vi "FocalMainV1.vi"() -> ()   [LabVIEW 2018]
uses:
  Clusters/FileDataChannel.ctl
  Clusters/BladePitchMode.ctl
  Clusters/GenMode.ctl
  Clusters/IndicatorScale.ctl
  Clusters/SimulationConstants.ctl
  <vilib>/Platform/TimedLoop/XDataNode/timing_clust.ctl
  <vilib>/Platform/TimedLoop/XDataNode/nitl_modes.ctl
  <vilib>/Platform/TimedLoop/XDataNode/wakeup.ctl
  Clusters/IOSignals.ctl
  Clusters/ArrayPairs.ctl
  Clusters/SwapArrayCluster.ctl
  Clusters/ElmoState.ctl
  Clusters/PLCSignals.ctl
  Clusters/CtrlSignals.ctl
  Clusters/ScalingEnum.ctl
  Clusters/RoscoParams.ctl
  Clusters/GenCtrl.ctl
  Clusters/PitchCtrl.ctl
  <vilib>/Utility/file.llb/Read Delimited Spreadsheet (DBL).vi
  SubVIs/InsertIntoArray_v2.vi
  <vilib>/platform/TimedLoop/XDataNode/XDataNode.xnode
  <vilib>/Platform/TimedLoop/XDataNode/XDNodeRunTimeDep.lvlib
  <resource>/objmgr/IndComECAT.rc
  usr/local/lib/libCallROSCO.so
panel:
  out "towerBotMy":dbl
  out "Current Setting":dbl[](array[numeric])
  in  "Commit":bool
  in  "Fan Setpoint (%)":dbl format="%#_13g"
  in  "Clear Faults":bool
  in  "Enable Fans":bool
  in  "Turn Fans On":bool
  out "Fy":dbl format="%#_5g"
  out "Fx":dbl
  out "PLC read errors":string
  out "PLC read/write late?":bool
  out "PLC Read Error":bool
  out "Axis 3 Homing":bool
  out "Axis 2 Homing":bool
  out "Axis 1 Homing":bool
  in  "Home Blades (x3)":bool
  out "Axis 3 Homed":bool
  out "Axis 2 Homed":bool
  out "Axis 1 Homed":bool
  out "SimulationConst":T1={"nGear"=1.0, "rotorRadius"=120.0, "numBlades"=3, "scaleFactor"=70.0, "roscoInitMinSpeed_rad_s"=0.5, "roscoInitMinTorqueFS_Nm"=1000000.0, "beckhoff24BitExt"=7812500, "torqueCellFullV"=5.0, "torqueCellFullNm"=2.0, "torqueCellELM3148V"=10.0, "nacelleAccELM3604V"=1.25, "nacelleAccScaleX"=0.0673, "nacelleAccOfstX"=0.0055, "nacelleAccScaleY"=0.0672, "nacelleAccOfstY"=0.0049, "nacelleAccScaleZ"=0.0677, "nacelleAccOfstZ"=0.0087, "cyberGearRatio"=0.5, "cyberLinesPerRev"=0.5, "cyberRatedTorque"=0.5, "towerTopForceScale"=0.5, "towerTopTorqueScale"=0.5, "plcSetpointScaling_norm2VFD"=0.5, "towerBotScaleMy_Nm_V"=0.5, "towerBotOfstMy_Nm"=0.5, "towerTopScaleXaxis_N_V"=0.5, "towerTopOfstXaxis_N"=0.5, "towerTopScaleYaxis_N_V"=0.5, "towerTopOfstYaxis_N"=0.5} {"beckhoff24BitExt" format="%x"}
  out "nacelleAccZ (m/s2)":dbl
  out "nacelleAccY (m/s2)":dbl
  out "nacelleAccX (m/s2)":dbl
  out "Disk > 2GB free?":bool
  out "Current OP mode":T2
  in  "IndicatorScale":T3
  in  "DISCON.IN file":string="DISCON-UMaineSemi.IN"
  in  "Cp/Ct/Cq file":string="Cp_Ct_Cq.IEA15MW.txt"
  out "Torque sine period FS (Nm)":dbl format="%.2g"
  out "Torque sine amp FS (Nm)":dbl format="%.2g"
  out "Torque sine mean FS (Nm)":dbl format="%.2g"
  out "Ramp time FS (s)":dbl format="%.2g"
  out "Ramp target vel FS (rpm)":dbl format="%.2g"
  out "Const. vel setpoint FS (rpm)":dbl format="%.2g"
  out "From File Vel FS (rpm)":dbl
  out "From File Pitch FS (deg)":dbl
  out "Exp time FS (s)":dbl format="%5.2f"
  in  "Commit get settings":bool
  out "Current OP mode":T4
  in  "Commit pitch settings":bool
  in  "Start / Stop Run":bool
  out "Speed Setpoint (rpm)":dbl(knob)=7.068579725455493e-05 scale=0.0..20.0
  out "Pitch Blade 3 (deg)":dbl
  out "Pitch Bade 2 (deg)":dbl
  out "Pitch Blade 1 (deg)":dbl
  out "Pitch Setpoint (deg)":dbl
  out "Setpoint file loaded":path
  in  "Setpoint file name":string="setpointsVelTestA.txt"
  out "Torque sine period MS (Nm)":dbl format="%.2g"
  out "Torque sine amp MS (Nm)":dbl format="%#.2g"
  in  "Torque sine period (s)":dbl=100.0
  in  "Torque sine amp (MNm)":dbl
  out "Torque sine mean MS (Nm)":dbl format="%.2g"
  in  "Torque mean (MNm)":dbl
  out "Ramp time MS (s)":dbl format="%.2g"
  out "Ramp target vel MS (rpm)":dbl format="%.2g"
  out "Const. vel setpoint MS (rpm)":dbl format="%.2g"
  in  "Ramp time (s)":dbl=100.0
  in  "Ramp target vel (rpm)":dbl=10.0
  in  "Const. vel (rpm)":dbl
  out "Current Const. (deg)":dbl
  in  "Next OP mode":T2
  in  "Next Const. (deg)":dbl=10.0
  in  "Next OP mode":T4
  in  "Wind Est. u(t=0)":dbl=5.0
  out "Exp. Time MS (s)":dbl format="%5.1f"
  out "Output file Name":string
  out "State logic late?":bool
  out "Axis 3 Fault":bool
  out "Axis 3 Warning":bool
  out "Axis 2 Fault":bool
  out "Axis 2 Warning":bool
  out "Axis 1 Fault":bool
  out "Axis 1 Warning":bool
  out "Axis 3 Operational":bool
  out "Axis 2 Operational":bool
  out "Axis 1 Operational":bool
  out "Pitch Axis 3 State":string
  out "Pitch Axis 2 State":string
  out "Pitch Axis 1 State":string
  in  "Clear Pitch Actuator Faults (x3)":bool
  in  "Enable Pitch Actuators (x3)":bool
  out "Generator Operational":bool
  in  "Clear Accelnet Faults":bool
  in  "Enable Accelnet":bool
  out "Generator Fault":bool
  out "Generator Warning":bool
  out "Main generator state":string
  out "Rosco Failed?":bool
  out "Torque Cell":dbl(knob) scale=0.0..25.0
  out "Actual Speed MS (rpm)":dbl(knob)=7.068579725455493e-05 scale=0.0..20.0
  in  "?":T5(tab)
  out "Generator Speed":dynamicdata(graph)
  out "Rotor Loads":dynamicdata(graph)
  out "Pitch":dynamicdata(graph)
  out "TSR":dynamicdata(graph)
  out "DISCON.IN Contents":string
  out "Rosco Interface Current Message":string
  out "ROSCO DISCON.In file used":string
  out "ROSCO CpCqCt File used":string
  out "ROSCO out file used":string
  out "Test sum":sgl
  out "error out":errorcluster
  out "aviFAIL":i32
  out "Rosco Interface First Message":string
  out "Rosco Setpoint (Nm) - MS":dbl(knob) scale=0.0..10.0
  out "OUT_ROTSP":dbl
  out "OUT_AEROTQ":dbl
  out "Rosco Pitch Setpoint (rad)":dbl(knob) scale=0.0..10.0
  out "WE ROSCO":dbl
  out "avrSWAP":sgl[](array[numeric])
  out "Setpoints":dbl[][](array[numeric])
  out "Time index":i32
  out "Loop duration (ms)":i64
  in  "Pitch Max Vel Change (rpm/min) - FS":dbl=10.0
  in  "Pitch Max Vel (rpm) - FS":dbl=1.0
  in  "Pitch Homing Vel  (rpm) - FS":dbl=0.3
  in  "Pitch P-Gain":dbl=5.0
  in  "Max Vel (rpm)  -FS":dbl=14.0
  in  "Velocity Ctrl P-Gain":dbl=0.14
  in  "Velocity Ctrl I-Gain":dbl=3.0
  in  "Torque Ctrl FF Gain":dbl=1.15
  in  "Torque Ctrl I-Gain":dbl=5.0
  in  "Torque Ctrl P-Gain":dbl=0.05
  in  "Max Torque (MNm) - FS":dbl=25.0
  out "Pitch axis 3 ctrl word":u16 format="%x"
  out "Pitch axis 2 ctrl word":u16 format="%x"
  out "RT Loop Duration":i64
  out "Control Mode - Main Gen":u8
  out "WriteSDO Abort - Main Gen":u32
  out "ReadSDO Abort - Main Gen":u32
  out "Gen ctrl word":u16 format="%x"
  out "Pitch axis 1 ctrl word":u16 format="%x"
  out "Graphics Update t (s)":dbl format="%.1f"
  out "Effective graphics rate (ms)":dbl format="%#.1f"
  out "WriteSDO Abort - Pitch 1":u32
  out "ReadSDO Abort - Pitch 1":u32
  out "Control Mode - Pitch 1":u8
  out "Torque RAW (V)":dbl
  out "Torque Sensor (Nm) - NOT scaled":dbl(knob) scale=-2.0..2.0
  out "Free GB disk":dbl
  out "WriteSDO Abort - Pitch 2":u32
  out "Control Mode - Pitch 2":u8
  out "ReadSDO Abort - Pitch 2":u32
  out "WriteSDO Abort - Pitch 3":u32
  out "Control Mode - Pitch 3":u8
  out "ReadSDO Abort - Pitch 3":u32
  out "MotorDemandTorque_Nm":dbl(knob) scale=-2.0..2.0
  out "MotorCurrentTorq (Nm)":dbl(knob) scale=-2.0..2.0
  out "Axis 1 HomePos (rad)":dbl
  out "Axis 2 HomePos (rad)":dbl
  out "Axis 3 HomePos (rad)":dbl
  out "TSR 2":dynamicdata(graph)
  out "Init error":errorcluster
  out "Torque Setpoint":dbl(knob) scale=0.0..35.0
  out "Power (MW)":dbl(slide) scale=0.0..10.0 scale format="%.2f"
  out "FIFO Loop Late?":bool
  in  "Base filename":string="rosco-tests"
  out "Writing":bool
  in  "?":T6
  out "#RT FIFO":u32
  in  "Stop LabVIEW":bool
  out "cRio Time(s)":dbl format="%6.1f"
  out "RT Loop Late?":bool
  # "FOCAL Campaign 1 - V1.0"
  # "ROSCO OK?"
  # "GENERATOR ENABLE"
  # "BLADE PITCH"
  # "WIND MACHINE CONTROL"
  # "EXPERIMENT CONTROL"
  # "GENERATOR SETPOINT CTRL"
  # "PITCH ACTUATORS CONTROL"
  # "Nacelle Acceleration"
  # "TowerTop 3DOF"
  # "Blade1"
  # "Blade2"
  # "Blade3"
  # "Current values"
  # "Operational"
  # "Enter NEXT values (FS)"
  # "FS"
  # "MS"
  # "Homing"
  # "Homed"
  # "Warning"
  # "Error"
  # "TowerBot My"
  # "Fan 1"
  # "Time"
  # "Pitch"
  # "Vel"
  # "Fan 20"
  # "Fan 30"
  # "Fan 10"
  # "PI for Torque Ctrl"
  # "PI for Velocity Ctrl"
  # "PI for Pitch Ctrl"
  # "Main Gen Limits"
  # "Pitch limits"
  # "PITCH AXIS 1"
  # "PITCH AXIS 2"
  # "PITCH AXIS 3"
  # "TOWER TOP 6DOF"
  # "SYSTEM"
  # "GENERATOR"
  # "TORQUE SENSOR"
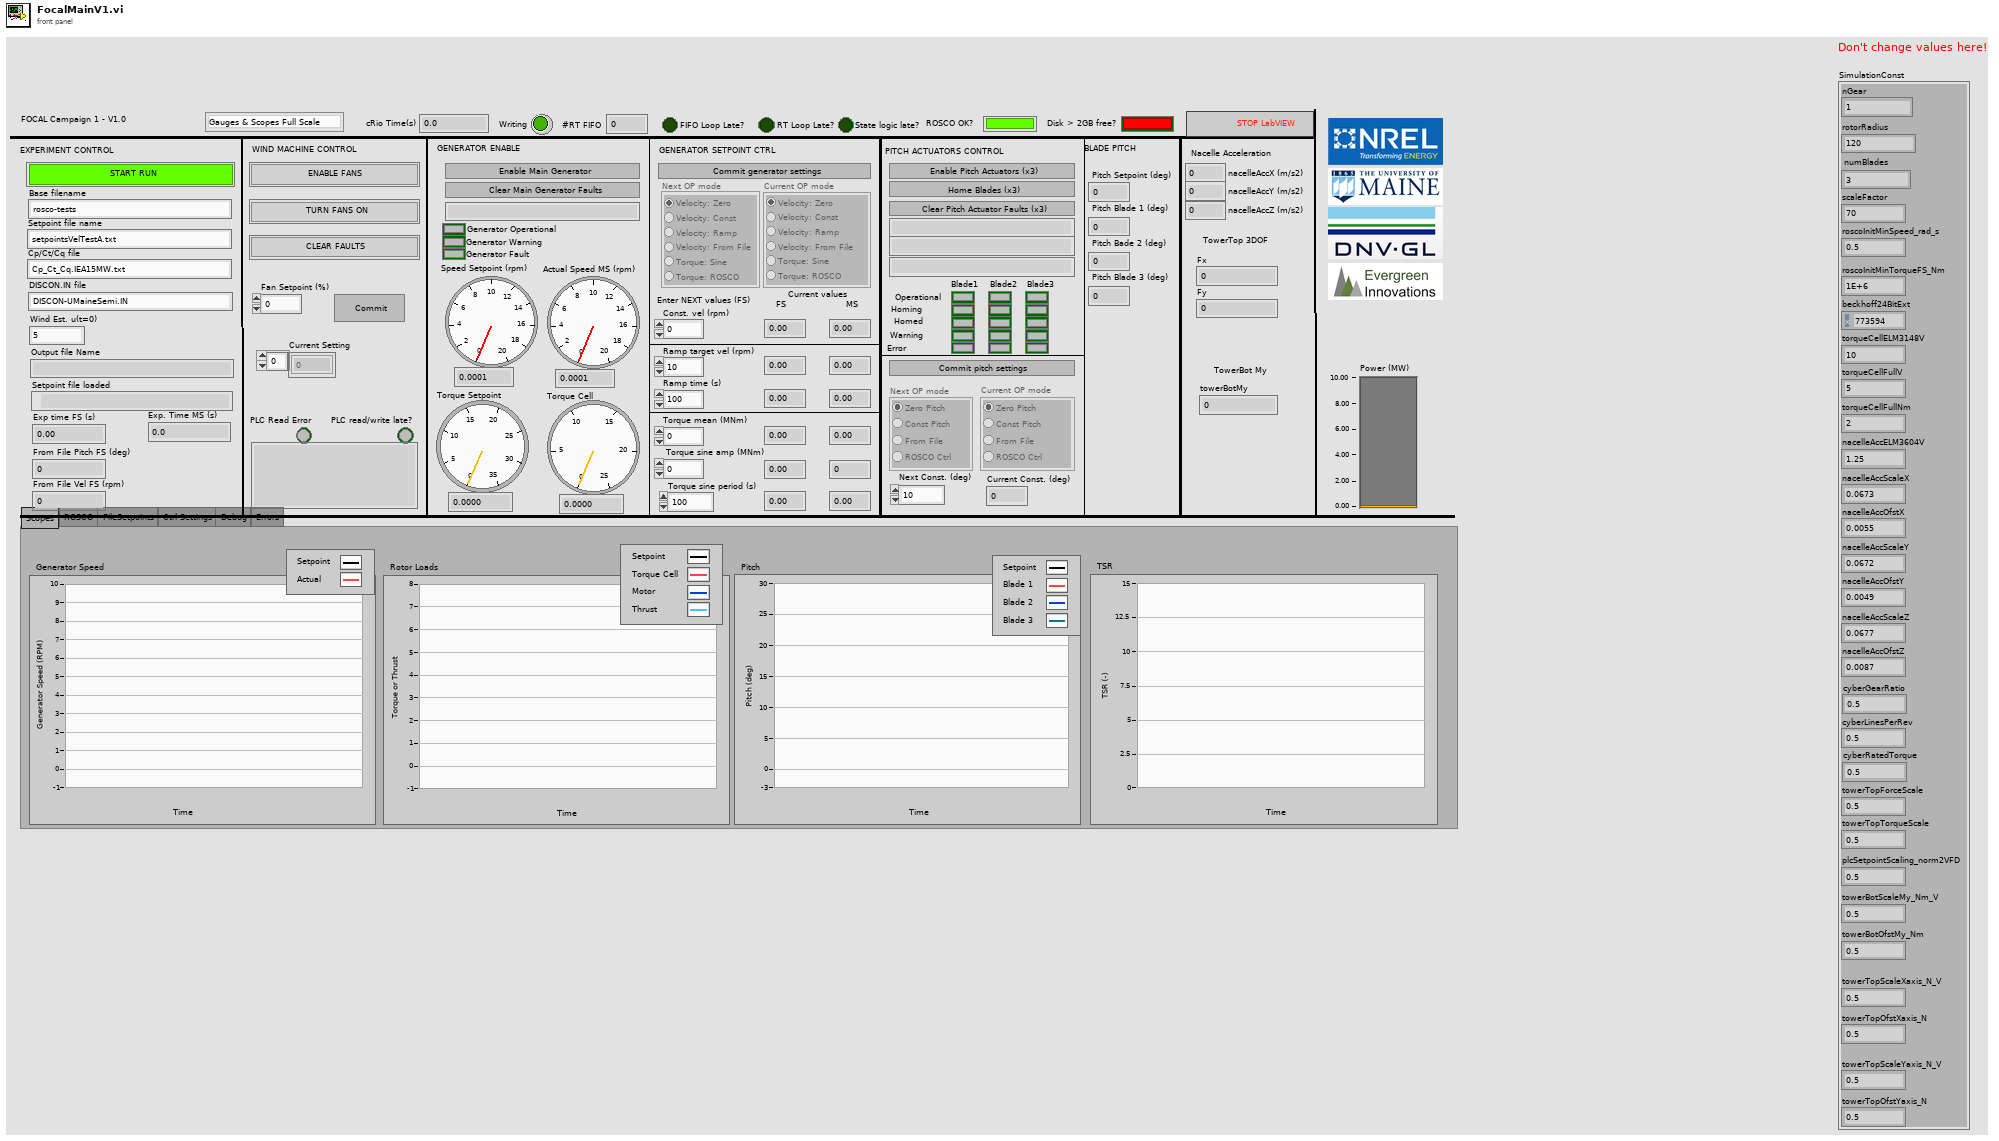
[diagram p1: front panel]
types:
  T1 = typedef "SimulationConstants.ctl" = cluster{"nGear":dbl, "rotorRadius":sgl, "numBlades":i32, "scaleFactor":dbl, "roscoInitMinSpeed_rad_s":dbl, "roscoInitMinTorqueFS_Nm":dbl, "beckhoff24BitExt":i32, "torqueCellFullV":dbl, "torqueCellFullNm":dbl, "torqueCellELM3148V":dbl, "nacelleAccELM3604V":dbl, "nacelleAccScaleX":dbl, "nacelleAccOfstX":dbl, "nacelleAccScaleY":dbl, "nacelleAccOfstY":dbl, "nacelleAccScaleZ":dbl, "nacelleAccOfstZ":dbl, "cyberGearRatio":dbl, "cyberLinesPerRev":dbl, "cyberRatedTorque":dbl, "towerTopForceScale":dbl, "towerTopTorqueScale":dbl, "plcSetpointScaling_norm2VFD":dbl, "towerBotScaleMy_Nm_V":dbl, "towerBotOfstMy_Nm":dbl, "towerTopScaleXaxis_N_V":dbl, "towerTopOfstXaxis_N":dbl, "towerTopScaleYaxis_N_V":dbl, "towerTopOfstYaxis_N":dbl}
  T2 = typedef "GenMode.ctl" = enum32{"Velocity: Zero", "Velocity: Const.", "Velocity: Ramp", "Velocity: From File", "Torque: Sine", "Torque: ROSCO"}
  T3 = typedef "IndicatorScale.ctl" = enum16{"Gauges & Scopes Full Scale", "Gauges & Scopes Model Scale"}
  T4 = typedef "BladePitchMode.ctl" = enum32{"Zero pitch", "Const pitch", "From File", "ROSCO Ctrl"}
  T5 = enum32{"Scopes", "ROSCO", "FileSetpoints", "Ctrl Settings", "Debug", "Errors"}
  T6 = typedef "FileDataChannel.ctl" = cluster{"dataTime_s":dbl, "dataLoopCounter":dbl, "genPosition_rad":dbl, "genSpeed_rad_s":dbl, "genTorque_Nm":dbl, "genStatus":dbl, "accelNacelleAx_m_s2":dbl, "accelNacelleAy_m_s2":dbl, "accelNacelleAz_m_s2":dbl, "pitch1Position_rad":dbl, "pitch1Velocity_rad_s":dbl, "pitch1Status":dbl, "pitch2Position_rad":dbl, "pitch2Velocity_rad_s":dbl, "pitch2Status":dbl, "pitch3Position_rad":dbl, "pitch3Velocity_rad_s":dbl, "pitch3Status":dbl, "torqueSetpointRosco_Nm":dbl, "pitchSetpointRosco_rad":dbl, "torqueSetpointActual_Nm":dbl, "pitchSetpointActual_rad":dbl, "velocitySetpoint_radps":dbl, "genUserOpMode":dbl, "pitchUserOpMode":dbl, "towerTopFx_N":dbl, "towerTopFy_N":dbl, "towerTopFz_N":dbl, "towerTopMx_Nm":dbl, "towerTopMy_Nm":dbl, "towerTopMz_Nm":dbl, "towerBotMy_Nm":dbl}
  T7 = typedef "CtrlSignals.ctl" = cluster{"Enable":bool, "On":bool, "Reset Fault":bool, "Velocity (VFD)":i32[]}
  T8 = typedef "PLCSignals.ctl" = cluster{"Enabled":bool[], "On":bool[], "Fault":bool[], "Velocity_VFD":i32[]}
  T9 = typedef "ElmoState.ctl" = cluster{"Elmo Operational":bool, "Elmo Warning":bool, "Elmo Fault":bool, "Blade Homed":bool, "Blade Homing":bool, "HomePos (rad)":dbl}
  T10 = typedef "ArrayPairs.ctl" = cluster{"iStatus":T11, "TIME":T11, "DT":T11, "Blade1PitchPos_rad":T11, "VS_MECHGENPWR":T11, "VS_GENPWR":T11, "GEN_SPEED":T11, "ROTOR_SPEED":T11, "GENTQMEAS":T11, "Y_M":T11, "HORWINDV":T11, "ROOTMOOP1":T11, "ROOTMOOP2":T11, "Blade2PitchPos_rad":T11, "Blade3PitchPos_rad":T11, "ROOTMOOP3":T11, "AVCMSG_SIZE":T11, "INFILE_SIZE ":T11, "OUTFILE_SIZE ":T11, "FA_ACC":T11, "NUM_BLADES":T11, "BladePitchSetpoint_rad":T11, "TorqueSetpoint_Nm":T11, "OUT_AEROTQ":T11, "Out.RotSpeed ":T11, "Out.DEBUG":T11}
  T11 = typedef "SwapArrayCluster.ctl" = cluster{"Index":i32, "Value":dbl}
  T12 = typedef "IOSignals.ctl" = cluster{"mainGenPosition (rad)":dbl, "motorCurrentTorq (Nm)":dbl, "mainGenVelocity (rad/s)":dbl, "mainGenStatus":u16, "pitch1Position (rad)":dbl, "pitch1Velocity (rad/s)":dbl, "pitch1Status":u16, "pitch2Position (rad)":dbl, "pitch2Velocity (rad/s)":dbl, "pitch2Status":u16, "pitch3Position (rad)":dbl, "pitch3Velocity (rad/s)":dbl, "pitch3Status":u16, "torqueSensor (Nm)":dbl, "nacelleAccX (m/s2)":dbl, "nacelleAccY (m/s2)":dbl, "nacelleAccZ (m/s2)":dbl, "pitch1HomeFlag":bool, "pitch2HomeFlag":bool, "pitch3HomeFlag":bool, "towerTopFx (N)":dbl, "towerTopFy (N)":dbl, "towerBotMy (Nm)":dbl}
  T13 = enum16{"open", "replace", "create", "open or create", "replace or create", "replace or create with confirmation"}
  T14 = typedef "RoscoParams.ctl" = cluster{"avrSWAP":dbl[], "aviFAIL":i32, "currentMsg":string, "ReturnValue":i32, "disconInFileName":string, "outFileName":string, "firstMsg":string}
  T15 = typedef "XDNodeRunTimeDep.lvlib/timing_clust.ctl" = cluster{"Expected End [f-1]":u64, "Actual End [f-1]":u64, "Finished Late? [f-1]":bool, "Expected End [i-1]":u64, "Actual End [i-1]":u64, "Finished Late? [i-1]":bool, "Expected Start [i]":u64, "Actual Start [i]":u64, "Expected Start [f]":u64, "Actual Start [f]":u64, "Source Name":string, "Structure Name":string, "Period":i64, "Deadline":i64, "Offset":i64, "Start":i64, "Priority":i32, "Timeout":i32, "Mode":T16, "Wakeup Reason":T17, "Error":errorcluster, "Source Type":string, "Secondary Source Type":string, "Global End Time":u64, "Global Start Time":u64, "Frame Duration":u64, "Iteration Duration":u64, "Assigned CPU":i32, "I/O Scan Engine Mode":u32}
  T16 = typedef "XDNodeRunTimeDep.lvlib/nitl_modes.ctl" = enum32{"No Change", "Process missed periods, maintain original phase", "Discard missed periods, maintain original phase", "Process missed periods, ignore original phase", "Discard missed periods, ignore original phase"}
  T17 = typedef "XDNodeRunTimeDep.lvlib/wakeup.ctl" = enum32{"Normal", "Aborted", "Asynchronous wakeup", "Timing source error", "Timed loop error", "Timeout"}
  T18 = typedef "ScalingEnum.ctl" = enum16{"Model scale -> Full scale", "Full scale -> Model scale"}
  T19 = typedef "GenCtrl.ctl" = cluster{"Constant velocity setpoint (rpm)":dbl, "Ramp target velocity (rpm)":dbl, "Ramp time (s)":dbl, "Sine mean (Nm)":dbl, "Sine amp (Nm)":dbl, "Sine period (s)":dbl, "Torque Ctrl I-Gain":dbl, "Velocity Ctrl P-Gain":dbl, "Velocity Ctrl I-Gain":dbl, "Max Torque (Nm)":dbl, "GeneratorOn":bool, "Torque Ctrl P-Gain":dbl, "From file velocity (rpm)":dbl, "Generator operating mode":T2, "Max Vel (rpm)":dbl, "Torque Ctrl FF Gain":dbl}
  T20 = typedef "PitchCtrl.ctl" = cluster{"P-Gain":dbl, "Blade pitch operating mode":T4, "Constant setpoint (deg)":dbl, "I-Gain":dbl, "Pitch from File (deg)":dbl, "Homing vel (rpm)":dbl, "Max vel (rpm)":dbl, "Max vel change (rpm/min)":dbl}
  T21 = typedef "AccelnetState.ctl" = cluster{"State String":string, "Accelnet Warning":bool, "Accelnet Fault":bool, "Accelnet Operational":bool}
  T22 = enum8{"Enabled", "Disabled", "Disabled and Grayed Out"}
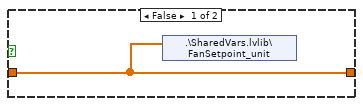
[diagram p3: hidden frame]
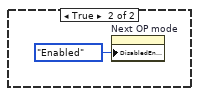
[diagram p10: hidden frame]
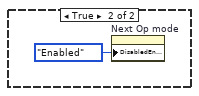
[diagram p11: hidden frame]
diagram:
  w3 = T8 {"Enabled"=[], "On"=[], "Fault"=[], "Velocity_VFD"=[]}  # PLCSignals
  w2 = errorcluster {"status"=FALSE, "code"=0, "source"=""}  # Error
  w46 = i64 1000 ("Period")
  # "Adjust this once we get a feeling for IO latency to/from the PLC"
  # "us -> s"
  # "in us"
  # "Init torque sine period"
  # "Init torque sine amp"
  # "Init torque mean"
  # "Init Ramp time"
  # "Init Ramp target vel"
  # "Init Const. Vel"
  # "Initial pitch"
  # "Code to remove"
  # "Vel"
  # "Pitch"
  # "Time"
  # "dt (s)"
  # "5ms = 200Hz"
  # "group name"
  n1 = flat-sequence {
    tunnel: [w95] -> w61
    tunnel: [w96] -> w60
    tunnel: [w88] -> w54
    tunnel: [w87] -> w53
    tunnel: [w74] -> w18
    tunnel: [w73] -> w17
    tunnel: [w72] -> w16
    tunnel: [w71] -> w15
    tunnel: w61 -> [w139]
    tunnel: w60 -> [w138]
    tunnel: w54 -> [w129]
    tunnel: w53 -> [w128]
    tunnel: [w125] -> w12
    tunnel: w18 -> [w116]
    tunnel: w17 -> [w115]
    tunnel: w16 -> [w105]
    tunnel: w15 -> [w104]
    tunnel: w12 -> [w149]
    tunnel: [w149] -> w11
    tunnel: [w205] -> w56
    tunnel: [w199] -> w64
    tunnel: [w190] -> w37
    tunnel: [w189] -> w30
    tunnel: [w187] -> w32
    tunnel: w11 -> [w187]
    tunnel: [w165] -> w20
    frame #0 {
      w72 = refnum<k21> "ni.var.io://NI-cRIO-9036-01B82934/EtherCAT Master/PitchBlade3" ("Slave Constant")
      w74 = refnum<k21> "ni.var.io://NI-cRIO-9036-01B82934/EtherCAT Master/PitchBlade2" ("Slave Constant")
      w88 = refnum<k21> "ni.var.io://NI-cRIO-9036-01B82934/EtherCAT Master/PitchBlade1" ("Slave Constant")
      w95 = refnum<k21> "ni.var.io://NI-cRIO-9036-01B82934/EtherCAT Master/MainGen" ("Slave Constant")
      # "Mode of operation for Pitch Blade 3"
      # "Mode of operation"
      # "8 = CSP \n9 = CSV\n10 = CST"
      # "Mode of operation for Pitch Blade 2"
      # "Mode of operation"
      # "8 = CSP \n9 = CSV\n10 = CST"
      # "Note: Operate in CST, and close velocity loop in LabVIEW when required"
      # "Mode of operation for Pitch Blade 1"
      # "Mode of operation for Main Gen"
      # "Mode of operation"
      # "8 = CSP \n9 = CSV\n10 = CST"
      # "Mode of operation"
      # "9 = CSV\n10 = CST"
      # "Set modes of operation for main generator and pitch actuators"
      n2 = invoke class="IndComECAT Slave" method="neLVRefNum_Slave_WriteSDO"(reference=w88, "Blocking"=TRUE, "OD Addr"=u16 0, "Index"=u16 24672, "Subindex"=u8 0, "Data"=u8[] [9]) -> (error out=w87:errorcluster, "Abort Code"=→"WriteSDO Abort - Pitch 1":u32)  [unwired: 3 in, 7 out]
      n3 = invoke class="IndComECAT Slave" method="neLVRefNum_Slave_WriteSDO"(reference=w74, "Blocking"=TRUE, "OD Addr"=u16 0, "Index"=u16 24672, "Subindex"=u8 0, "Data"=u8[] [9]) -> (error out=w73:errorcluster, "Abort Code"=→"WriteSDO Abort - Pitch 2":u32)  [unwired: 3 in, 7 out]
      n4 = invoke class="IndComECAT Slave" method="neLVRefNum_Slave_WriteSDO"(reference=w95, "Blocking"=TRUE, "OD Addr"=u16 0, "Index"=u16 24672, "Subindex"=u8 0, "Data"=u8[] [10]) -> (error out=w96:errorcluster, "Abort Code"=→"WriteSDO Abort - Main Gen":u32)  [unwired: 3 in, 7 out]
      n5 = invoke class="IndComECAT Slave" method="neLVRefNum_Slave_WriteSDO"(reference=w72, "Blocking"=TRUE, "OD Addr"=u16 0, "Index"=u16 24672, "Subindex"=u8 0, "Data"=u8[] [9]) -> (error out=w71:errorcluster, "Abort Code"=→"WriteSDO Abort - Pitch 3":u32)  [unwired: 3 in, 7 out]
    }
    frame #1 {
      # "Mode of operation"
      # "Mode of operation"
      # "Mode of operation"
      # "Mode of operation"
      # "Check generator and pitch actuator control modes"
      n6 = invoke class="IndComECAT Slave" method="neLVRefNum_Slave_ReadSDO"(reference=w139, error in=w138, "blocking"=TRUE, "odAddr"=u16 0 ("OD address"), "index"=u16 24672 ("Index"), "subIndex"=u8 0 ("Subindex")) -> (error out=w127:errorcluster, "data"=w142:u8[], "abortCode"=→"ReadSDO Abort - Main Gen":u32)  [unwired: 3 in, 6 out]
      n7 = invoke class="IndComECAT Slave" method="neLVRefNum_Slave_ReadSDO"(reference=w116, error in=w115, "blocking"=TRUE, "odAddr"=u16 0 ("OD address"), "index"=u16 24672 ("Index"), "subIndex"=u8 0 ("Subindex")) -> (error out=w114:errorcluster, "data"=w122:u8[], "abortCode"=→"ReadSDO Abort - Pitch 2":u32)  [unwired: 3 in, 6 out]
      n8 = invoke class="IndComECAT Slave" method="neLVRefNum_Slave_ReadSDO"(reference=w105, error in=w104, "blocking"=TRUE, "odAddr"=u16 0 ("OD address"), "index"=u16 24672 ("Index"), "subIndex"=u8 0 ("Subindex")) -> (error out=w103:errorcluster, "data"=w108:u8[], "abortCode"=→"ReadSDO Abort - Pitch 3":u32)  [unwired: 3 in, 6 out]
      n9 = invoke class="IndComECAT Slave" method="neLVRefNum_Slave_ReadSDO"(reference=w129, error in=w128, "blocking"=TRUE, "odAddr"=u16 0 ("OD address"), "index"=u16 24672 ("Index"), "subIndex"=u8 0 ("Subindex")) -> (error out=w126:errorcluster, "data"=w132:u8[], "abortCode"=→"ReadSDO Abort - Pitch 1":u32)  [unwired: 3 in, 6 out]
      n10 = Index Array(array=w142, index=0) -> (element=→"Control Mode - Main Gen":u8)
      n11 = Index Array(array=w122, index=0) -> (element=→"Control Mode - Pitch 2":u8)
      n12 = Index Array(array=w108, index=0) -> (element=→"Control Mode - Pitch 3":u8)
      n13 = Index Array(array=w132, index=0) -> (element=→"Control Mode - Pitch 1":u8)
      n14 = Merge Errors(w127, w126, w114, w103) -> (w125:errorcluster)
    }
    frame #2 {
      w148 = T1 {"nGear"=1.0, "rotorRadius"=120.0, "numBlades"=3, "scaleFactor"=70.0, "roscoInitMinSpeed_rad_s"=0.5, "roscoInitMinTorqueFS_Nm"=1000000.0, "beckhoff24BitExt"=7812500, "torqueCellFullV"=5.0, "torqueCellFullNm"=5.0, "torqueCellELM3148V"=10.0, "nacelleAccELM3604V"=1.25, "nacelleAccScaleX"=14.859, "nacelleAccOfstX"=0.0055, "nacelleAccScaleY"=14.881, "nacelleAccOfstY"=0.0049, "nacelleAccScaleZ"=14.771, "nacelleAccOfstZ"=0.0087, "cyberGearRatio"=64.0, "cyberLinesPerRev"=4096.0, "cyberRatedTorque"=5.1, "towerTopForceScale"=0.5, "towerTopTorqueScale"=0.5, "plcSetpointScaling_norm2VFD"=6000.0, "towerBotScaleMy_Nm_V"=193163.0, "towerBotOfstMy_Nm"=-0.0231, "towerTopScaleXaxis_N_V"=1.0, "towerTopOfstXaxis_N"=0.0, "towerTopScaleYaxis_N_V"=1.0, "towerTopOfstYaxis_N"=0.0} ("SimulationConst")
      # "Note:\nnacelleAcc constants are inverted from manufacturer sheets due to how we apply scale"
      # "Define constants to be used in the code"
      # "Define constants"
      n15 = shared-variable ".\\SharedVars.lvlib\\Const"(w148) -> ()  [unwired: 1 in, 1 out]
      "SimulationConst" <- w148
    }
    frame #3 {
      w177 = path "C:/rosco-data" ("path")
      # "This file will be picked up via DISCON.IN / ROSCO"
      # "Checks if DISCON.IN exists"
      # "Allocate memory for ROSCO return message"
      # "Up to 500 entries in SWAP array"
      # "No. of buffer slices"
      # "This is the typedef for File IO"
      # "number of channels"
      # "Read required files and initialize various arrays"
      n16 = disable-structure shown="Disabled" {
        frame Disabled {
          # "Note: DO NOT run this code in normal operation. Will  cause the .so file to not unload properly."
          # "Test function into libCallROSCO"
          n17 = dll-call lib="usr/local/lib/libCallROSCO.so" fn="add"("a"=sgl 1.0, "b"=sgl 8.0) -> (error out=→"error out":errorcluster, "sum"=→"Test sum":sgl)  [unwired: 5 in, 1 out]
        }
        frame Enabled {
        }
      }
      n18 = property on="Base filename" class="Str"("Value"="focal_series_000" ("Base filename")) -> ()  [unwired: 2 in, 2 out]
      n19 = property on="Rosco Interface Current Message" class="Str"("Value"="") -> ()  [unwired: 2 in, 2 out]
      n20 = property on="Base filename" class="Str"("Value"="") -> ()  [unwired: 2 in, 2 out]
      n21 = property on="StopLabVIEW" class="Bool (strict)"("Value"=FALSE) -> ()  [unwired: 2 in, 2 out]
      n22 = property on="Enable Accelnet" class="Bool (strict)"("Value"=FALSE ("Enable Accelnet")) -> ()  [unwired: 2 in, 2 out]
      n23 = property on="Enable Pitch Actuators (x3)" class="Bool (strict)"("Value"=FALSE ("Enable Pitch Actuators (x3)")) -> ()  [unwired: 2 in, 2 out]
      n24 = property on="Next Op mode" class="RadioBtnsControl (strict)"("Value"=GenMode."Velocity: Zero" ("Next Op mode")) -> ()  [unwired: 2 in, 2 out]
      n25 = property on="Next OP mode" class="RadioBtnsControl (strict)"("Value"=BladePitchMode."Zero pitch" ("Next OP mode")) -> ()  [unwired: 2 in, 2 out]
      n26 = Build Path(base path=path "C:/setpoints" ("file path (dialog if empty)"), name or relative path="Setpoint file name") -> (appended path=w184:path)
      n27 = Build Path(base path=w177, name or relative path="roscoOut.txt") -> (appended path=w175:path)
      n28 = Build Path(base path=w177, name or relative path="Cp/Ct/Cq file") -> (appended path=w182:path)
      n29 = Build Path(base path=w177, name or relative path="DISCON.IN file") -> (appended path=w178:path)
      n30 = call "ConfigFileExists.vi"("Path   In"=w184) -> ("Path Out"=w188:path)  [unwired: 10 in]
      "Setpoint file loaded" <- w188
      n31 = call "ConfigFileExists.vi"("Path   In"=w178) -> ("Path Out"=w171:path)  [unwired: 10 in]
      n32 = call "ConfigFileExists.vi"("Path   In"=w182) -> ("Path Out"=w181:path)  [unwired: 10 in]
      n33 = Path To String(path=w175) -> (string=w174:string)
      "ROSCO out file used" <- w174
      n34 = Path To String(path=w181) -> (string=→"ROSCO CpCqCt File used":string)
      n35 = Path To String(path=w171) -> (string=w173:string)
      "ROSCO DISCON.In file used" <- w173
      n36 = call-poly <vilib>:"Read Delimited Spreadsheet.vi"("file path (dialog if empty)"=w188, "format (%.3f)"="%.6f", "number of rows (all:-1)"=-1) -> ("all rows"=w190:dbl[][], "error out"=w189:errorcluster)  [unwired: 7 in, 4 out]
      n37 = Open/Create/Replace File(file path (use dialog)=w171, operation (0:open)=T13."open") -> (refnum out=w169:refnum<file>, error out=w172:errorcluster)  [unwired: 4 in, 1 out]
      n38 = property on="Velocity Ctrl P-Gain" class="DigNum (strict)"("Value"=0.05 ("Velocity Ctrl P-Gain")) -> ()  [unwired: 2 in, 2 out]
      n39 = property on="Velocity Ctrl I-Gain" class="DigNum (strict)"("Value"=7.0 ("Velocity Ctrl I-Gain")) -> ()  [unwired: 2 in, 2 out]
      n40 = property on="Max Torque (MNm) - FS" class="DigNum (strict)"("Value"=25.0 ("Max Torque (MNm) - FS")) -> ()  [unwired: 2 in, 2 out]
      n41 = property on="Max Vel (rpm)  -FS" class="DigNum (strict)"("Value"=15.0 ("Max Vel (rpm)  -FS")) -> ()  [unwired: 2 in, 2 out]
      n42 = property on="Torque Ctrl P-Gain" class="DigNum (strict)"("Value"=0.05 ("Torque Ctrl P-Gain")) -> ()  [unwired: 2 in, 2 out]
      n43 = property on="Torque Ctrl I-Gain" class="DigNum (strict)"("Value"=10.0 ("Torque Ctrl I-Gain")) -> ()  [unwired: 2 in, 2 out]
      n44 = property on="Torque Ctrl FF Gain" class="DigNum (strict)"("Value"=1.25 ("Torque Ctrl FF Gain")) -> ()  [unwired: 2 in, 2 out]
      n45 = call "StringInit.vi"("accOUTNAME"="First Msg", "dimension size"=8192) -> ("result string"=w161:string)  [unwired: 9 in]
      n46 = call "StringInit.vi"("accOUTNAME"="Current Msg", "dimension size"=8192) -> ("result string"=w164:string)  [unwired: 9 in]
      n47 = Initialize Array(0.0 ("element"), 500 ("dimension size")) -> (w197:dbl[])
      n48 = Read from Text File(file (use dialog)=w169, error in=w172) -> (refnum out=w167:refnum<file>, text=→"DISCON.IN Contents":string, error out=w166:errorcluster)  [unwired: 2 in, 1 out]
      n49 = Close File(refnum=w167, error in=w166) -> (error out=w165:errorcluster)  [unwired: 1 out]
      n50 = Bundle By Name(cluster=T14 {"avrSWAP"=[], "aviFAIL"=0, "currentMsg"="", "ReturnValue"=0, "disconInFileName"="", "outFileName"="", "firstMsg"=""}, "avrSWAP"=w197, "aviFAIL"=-100, "currentMsg"=w164, "firstMsg"=w161, "outFileName"=w174, "disconInFileName"=w173) -> (w199:T14)
      n51 = Cluster To Array(cluster="?") -> (array=w195:dbl[])
      n52 = Array Size(array=w195) -> (size(s)=w194:i32)
      n53 = To Unsigned Long Integer(number=w194) -> (unsigned 32bit integer=w193:u32)
      n54 = RT FIFO Create(0:"DataBuffer" ("name (unnamed)"), 1:dbl[] [] ("appended array"), 4:u32 200, 6:w193) -> (8:w205:refnum<k33>)  [unwired: 4 in, 2 out]
    }
  }
  n55 = disable-structure shown="Disabled" {
    frame Disabled {
      n56 = shared-variable ".\\SharedVars.lvlib\\SIM-GenSpeed_rad_s"(0.009999999776482582 ("RotorSpeed(rad/s)")) -> ()  [unwired: 1 in, 1 out]
      n57 = shared-variable ".\\SharedVars.lvlib\\SIM-BladePitch_rad"(0.0 ("ecat-BladePitch")) -> ()  [unwired: 1 in, 1 out]
      n58 = shared-variable ".\\SharedVars.lvlib\\SIM-WindSpeed_m_s"(0.0 ("WindSpeedSim")) -> ()  [unwired: 1 in, 1 out]
    }
    frame Enabled {
    }
  }
  n59 = disable-structure shown="Disabled" {
    frame Disabled {
      n60 = local read "DISCON.IN Contents"() -> ()  [unwired: 1 in]
    }
    frame Enabled {
    }
  }
  n61 = Merge Errors(w20, w32, w30) -> (→"Init error":errorcluster)
  n62 = property on="SimulationConst" class="Clust (strict)"() -> ("Controls[]"=w10:refnum<vi>[])  [unwired: 2 in, 2 out]
  n63 = for {
    tunnel: w10 -> [w223] mode=indexing
    tunnel: [w224] -> w14 mode=indexing
    tunnel: [w220] -> w13 mode=indexing
    n64 = property class="Ctl"(reference=w223) -> ("Value"=w222:variant)  [unwired: 1 in, 2 out]
    n65 = property class="Ctl"(reference=w223) -> ("Label.Text"=w224:string)  [unwired: 1 in, 2 out]
    n66 = Variant To Data(type=0.0, Variant=w222) -> (data=w220:dbl)  [unwired: 1 in, 1 out]
  }
  n67 = Tick Count (ms)() -> (millisecond timer value=w55:u32)
  n68 = property class="Clust (strict)"() -> ("Controls[]"=w70:refnum<vi>[])  [unwired: 2 in, 2 out]
  n69 = To Double Precision Float(number=w46) -> (double precision float=w45:dbl)
  n70 = for {
    tunnel: w70 -> [w226] mode=indexing
    tunnel: [w225] -> w69 mode=indexing
    n71 = property class="Ctl"(reference=w226) -> ("Label.Text"=w225:string)  [unwired: 1 in, 2 out]
  }
  n72 = Divide(x=w45, y=1000000.0) -> (x/y=w44:dbl)
  n73 = node-c288(i64 50 ("Period")) -> (w43:T15)  [unwired: 3 in]
  n74 = node-c288(i64 200 ("Period")) -> (w6:T15)  [unwired: 3 in]
  n75 = node-c288(w46) -> (w52:T15)  [unwired: 3 in]
  n76 = node-c288(i64 1 ("Period")) -> (w63:T15)  [unwired: 3 in]
  n77 = node-c288(i64 5 ("Period")) -> (w59:T15)  [unwired: 3 in]
  n78 = Index Array(array=w37, index (col)=0 ("disabled index (col)")) -> (element=w35:dbl[])  [unwired: 1 in]
  n79 = Index Array(array=w37, index (col)=1 ("disabled index (col)")) -> (element=w36:dbl[])  [unwired: 1 in]
  n80 = Index Array(array=w37, index (col)=2 ("disabled index (col)")) -> (element=w34:dbl[])  [unwired: 1 in]
  n81 = timed-loop {
    timing: w43 -> [_]
    timing-out: [_] -> w42
    tunnel: w36 -> [w303]
    tunnel: w35 -> [w305]
    tunnel: w34 -> [w302]
    shift-right: [w281] -> _
    shift-left: BladePitchMode."Zero pitch" ("PitchCtrlMode") -> [w298]
    shift-right: [w282] -> _
    shift-left: 0.0 -> [w296]
    shift-right: [w237] -> _
    shift-left: GenMode."Velocity: Zero" ("GenOpMode") -> [w294]
    shift-right: [w257] -> _
    shift-left: 0.0 -> [w267]
    shift-right: [w255] -> _
    shift-left: 5.0 -> [w266]
    shift-right: [w254] -> _
    shift-left: 100.0 -> [w265]
    shift-right: [w250] -> _
    shift-left: 0.0 -> [w264]
    shift-right: [w249] -> _
    shift-left: 0.0 -> [w263]
    shift-right: [w248] -> _
    shift-left: 0.0 -> [w262]
    shift-right: [w228] -> _
    shift-left: _ -> [w227]
    stop <- w310 stop-if-true
    w252 = 1000000.0 ("y")
    w280 = T19 {"Constant velocity setpoint (rpm)"=0.0, "Ramp target velocity (rpm)"=0.0, "Ramp time (s)"=0.0, "Sine mean (Nm)"=0.0, "Sine amp (Nm)"=0.0, "Sine period (s)"=0.0, "Torque Ctrl I-Gain"=0.0, "Velocity Ctrl P-Gain"=0.0, "Velocity Ctrl I-Gain"=0.0, "Max Torque (Nm)"=0.0, "GeneratorOn"=FALSE, "Torque Ctrl P-Gain"=0.0, "From file velocity (rpm)"=0.0, "Generator operating mode"=enum."Velocity: Zero", "Max Vel (rpm)"=0.0, "Torque Ctrl FF Gain"=0.0}  # Gen Control
    w285 = T20 {"P-Gain"=0.0, "Blade pitch operating mode"=enum."From File", "Constant setpoint (deg)"=0.0, "I-Gain"=0.0, "Pitch from File (deg)"=0.0, "Homing vel (rpm)"=0.0, "Max vel (rpm)"=0.0, "Max vel change (rpm/min)"=0.0}  # PitchCtrl
    # "Probably not required, but leave in cluster if needed"
    # "This code finds the NEAREST LOWER time. For example, if elements 40s and 50s exist in the input time vector, and tnow = 49s, the code will find the index for 40s."
    # "MNm-> Nm"
    # "Scale right after user input"
    # "Scale right after user input"
    # "MNm-> Nm"
    # "File setpoint and mode loop (RT, but only at 50 ms)"
    n82 = node-c288() -> (→"Loop duration (ms)":i64)  [unwired: 1 in]
    n83 = shared-variable ".\\SharedVars.lvlib\\ExpTime_s"() -> (w309:dbl)  [unwired: 1 in, 1 out]
    n84 = shared-variable ".\\SharedVars.lvlib\\Const"() -> (w308:T1)  [unwired: 1 in, 1 out]
    n85 = Unbundle By Name(w308) -> ("scaleFactor"=w307:dbl)
    n86 = case shown="True" "Commit" {
      tunnel: [w311 w314] -> w228
      tunnel: w227 -> [w311 _]
      frame False {
        n87 = shared-variable ".\\SharedVars.lvlib\\FanSetpoint_unit"(w311) -> ()  [unwired: 1 in, 1 out]
      }
      frame True {
        # "% to [0-1]"
        n88 = Divide(x="Fan Setpoint (%)", y=100.0) -> (x/y=w313:dbl)
        n89 = Initialize Array(w313, 32 ("dimension size")) -> (w314:dbl[])
        n90 = shared-variable ".\\SharedVars.lvlib\\FanSetpoint_unit"(w314) -> ()  [unwired: 1 in, 1 out]
      }
    }
    "Current Setting" <- w228
    n91 = case shown="True" "Commit get settings" {
      tunnel: w294 -> [w334 _]
      tunnel: [w334 w341] -> w236
      tunnel: "Next OP mode" -> [_ w341]
      tunnel: "Const. vel (rpm)" -> [_ w340]
      tunnel: "Ramp target vel (rpm)" -> [_ w339]
      tunnel: "Ramp time (s)" -> [_ w338]
      tunnel: "Torque mean (MNm)" -> [_ w337]
      tunnel: "Torque sine amp (MNm)" -> [_ w336]
      tunnel: "Torque sine period (s)" -> [_ w335]
      tunnel: w267 -> [w333 _]
      tunnel: w266 -> [w332 _]
      tunnel: w265 -> [w331 _]
      tunnel: w264 -> [w330 _]
      tunnel: w263 -> [w329 _]
      tunnel: w262 -> [w328 _]
      tunnel: [w333 w340] -> w257
      tunnel: [w332 w339] -> w255
      tunnel: [w331 w338] -> w254
      tunnel: [w330 w337] -> w250
      tunnel: [w329 w336] -> w249
      tunnel: [w328 w335] -> w248
      frame False {
      }
      frame True {
      }
    }
    n92 = shared-variable ".\\SharedVars.lvlib\\GeneratorOn"() -> (w238:bool)  [unwired: 1 in, 1 out]
    n93 = call "ScaleTime.vi"("Scale Dir"=ScalingEnum."Model scale -> Full scale", "Scale factor"=w307, "Time (In)"=w309) -> ("Time OUT (Out)"=w304:dbl)  [unwired: 8 in]
    "Exp time FS (s)" <- w304
    n94 = case shown="True" "Commit pitch settings" {
      tunnel: w298 -> [w343 _]
      tunnel: [w343 w345] -> w281
      tunnel: "Next OP mode" -> [_ w345]
      tunnel: w296 -> [w342 _]
      tunnel: [w342 w344] -> w282
      tunnel: "Next Const. (deg)" -> [_ w344]
      frame False {
      }
      frame True {
      }
    }
    n95 = Subtract(x=w305, y=w304) -> (x-y=w243:dbl[])
    n96 = Array Size(array=w243) -> (size(s)=w244:i32)
    n97 = Less Or Equal To 0?(x=w243) -> (x <= 0?=w245:bool[])
    n98 = case shown="False" w238 {
      tunnel: [GenMode."Velocity: Zero" ("Next OP mode") w318] -> w237
      tunnel: w236 -> [_ w318]
      frame False {
      }
      frame True {
      }
    }
    n99 = for {
      N: w244 -> [_]
      tunnel: w245 -> [w322] mode=indexing
      shift-right: [w319] -> w242
      shift-left: w243 -> [w321]
      i -> [w320]
      n100 = case shown="False" w322 {
        tunnel: w321 -> [w326 w327]
        tunnel: w320 -> [w325 _]
        tunnel: [w323 w327] -> w319
        frame False {
          n101 = Replace Array Subset(array=w326, new element=nan ("new element/subarray"), index=w325) -> (w323:dbl[])
        }
        frame True {
        }
      }
    }
    n102 = shared-variable ".\\SharedVars.lvlib\\FromFileVelFS_rpm"() -> (w274:dbl)  [unwired: 1 in, 1 out]
    n103 = shared-variable ".\\SharedVars.lvlib\\GeneratorOn"() -> (w272:bool)  [unwired: 1 in, 1 out]
    n104 = shared-variable ".\\SharedVars.lvlib\\FromFilePitchFS_deg"() -> (w283:dbl)  [unwired: 1 in, 1 out]
    n105 = Absolute Value(x=w242) -> (abs(x)=w241:dbl[])
    n106 = Array Max & Min(array=w241) -> (min index (indices)=w240:i32)  [unwired: 3 out]
    "Time index" <- w240
    n107 = Multiply(x=1000000.0 ("y"), y="Max Torque (MNm) - FS") -> (x*y=w278:dbl)
    n108 = Multiply(x=w252, y=w250) -> (x*y=w253:dbl)
    n109 = Multiply(x=w249, y=w252) -> (x*y=w251:dbl)
    n110 = shared-variable ".\\SharedVars.lvlib\\Const"() -> (w234:T1)  [unwired: 1 in, 1 out]
    n111 = shared-variable ".\\SharedVars.lvlib\\Const"() -> (w271:T1)  [unwired: 1 in, 1 out]
    n112 = Bundle By Name(cluster=w285, "Blade pitch operating mode"=w281, "P-Gain"="Pitch P-Gain", "I-Gain"=0.0, "Constant setpoint (deg)"=w282, "Pitch from File (deg)"=w283, "Homing vel (rpm)"="Pitch Homing Vel  (rpm) - FS", "Max vel (rpm)"="Pitch Max Vel (rpm) - FS", "Max vel change (rpm/min)"="Pitch Max Vel Change (rpm/min) - FS") -> (w258:T20)
    n113 = Bundle By Name(cluster=w280, "Sine period (s)"=w248, "Sine amp (Nm)"=w251, "Sine mean (Nm)"=w253, "Ramp time (s)"=w254, "Ramp target velocity (rpm)"=w255, "Constant velocity setpoint (rpm)"=w257, "Generator operating mode"=w237, "GeneratorOn"=w272, "From file velocity (rpm)"=w274, "Max Torque (Nm)"=w278, "Max Vel (rpm)"="Max Vel (rpm)  -FS", "Torque Ctrl P-Gain"="Torque Ctrl P-Gain", "Torque Ctrl I-Gain"="Torque Ctrl I-Gain", "Torque Ctrl FF Gain"="Torque Ctrl FF Gain", "Velocity Ctrl P-Gain"="Velocity Ctrl P-Gain", "Velocity Ctrl I-Gain"="Velocity Ctrl I-Gain") -> (w256:T19)
    n114 = Index Array(array=w303, index=w240) -> (element=w301:dbl)
    "From File Pitch FS (deg)" <- w301
    n115 = Index Array(array=w302, index=w240) -> (element=w300:dbl)
    "From File Vel FS (rpm)" <- w300
    n116 = Unbundle By Name(w234) -> ("scaleFactor"=w259:dbl)
    n117 = shared-variable ".\\SharedVars.lvlib\\FromFileVelFS_rpm"(w300) -> ()  [unwired: 1 in, 1 out]
    n118 = shared-variable ".\\SharedVars.lvlib\\FromFilePitchFS_deg"(w301) -> ()  [unwired: 1 in, 1 out]
    n119 = Unbundle By Name(w271) -> ("scaleFactor"=w270:dbl)
    n120 = call "ScalePitchCtrl.vi"("Scale Direction"=ScalingEnum."Full scale -> Model scale", "Scale Factor"=w259, "PitchCtrl (In)"=w258) -> ("PitchCtrl (Out)"=w261:T20)  [unwired: 8 in]
    n121 = shared-variable ".\\SharedVars.lvlib\\StopLabVIEW"() -> (w310:bool)  [unwired: 1 in, 1 out]
    n122 = call "ScaleGenCtrl.vi"("Scale Dir"=ScalingEnum."Full scale -> Model scale", "Scale factor"=w270, "Gen Control (In)"=w256) -> ("Gen Control (Out)"=w268:T19)  [unwired: 8 in]
    n123 = shared-variable ".\\SharedVars.lvlib\\PitchCtrlFS"(w258) -> ()  [unwired: 1 in, 1 out]
    n124 = shared-variable ".\\SharedVars.lvlib\\PitchCtrlMS"(w261) -> ()  [unwired: 1 in, 1 out]
    n125 = shared-variable ".\\SharedVars.lvlib\\GenCtrlFS"(w256) -> ()  [unwired: 1 in, 1 out]
    n126 = shared-variable ".\\SharedVars.lvlib\\GenCtrlMS"(w268) -> ()  [unwired: 1 in, 1 out]
    n127 = node-c288() -> ()  [unwired: 1 in, 1 out]
  }
  n128 = timed-loop {
    timing: w6 -> [_]
    timing-out: [_] -> w5
    shift-right: [w355] -> _
    shift-left: w3 -> [w358]
    tunnel: w2 -> [w360]
    tunnel: [w356] -> _
    stop <- w352 stop-if-true
    w353 = "192.168.1.52"  # PLC IP address
    # "192.168.1.52"
    # "Loop to update the PLC read / write tags"
    n129 = node-c288() -> (→"PLC read/write late?":bool)  [unwired: 1 in]
    n130 = call "ReadPLC.vi"("PC IP address"=w353, "Error In"=w360, "PLCSignals In"=w358) -> ("Error Out"=w357:errorcluster, "PLCSignals Out"=w354:T8, "Read errors"=→"PLC read errors":string, "Read Error"=→"PLC Read Error":bool)  [unwired: 5 in]
    n131 = shared-variable ".\\SharedVars.lvlib\\PLCCtrlSignals"() -> (w349:T7)  [unwired: 1 in, 1 out]
    n132 = shared-variable ".\\SharedVars.lvlib\\PLCInputSignals"(w354) -> ()  [unwired: 1 in, 1 out]
    n133 = call "WritePLC.vi"("Ctrl Signals"=w349, "PLC IP address"=w353, "Error In"=w357, "PLCSignals In"=w354) -> ("Error Out"=w356:errorcluster, "PLCSignals Out"=w355:T8)  [unwired: 6 in]
    n134 = shared-variable ".\\SharedVars.lvlib\\StopLabVIEW"() -> (w352:bool)  [unwired: 1 in, 1 out]
    n135 = node-c288() -> ()  [unwired: 1 in, 1 out]
  }
  n136 = timed-loop {
    timing: w52 -> [_]
    timing-out: [_] -> w51
    shift-right: [w384] -> _
    shift-left: w64 -> [w412]
    shift-right: [w368] -> w49
    shift-left: errorcluster {"status"=FALSE, "code"=0, "source"=""} ("error out") -> [w411]
    shift-right: [w385] -> _
    shift-left: T10 {"iStatus"={"Index"=0, "Value"=0.0}, "TIME"={"Index"=1, "Value"=0.0}, "DT"={"Index"=2, "Value"=0.0}, "Blade1PitchPos_rad"={"Index"=3, "Value"=0.0}, "VS_MECHGENPWR"={"Index"=13, "Value"=0.0}, "VS_GENPWR"={"Index"=14, "Value"=0.0}, "GEN_SPEED"={"Index"=19, "Value"=0.0}, "ROTOR_SPEED"={"Index"=20, "Value"=0.0}, "GENTQMEAS"={"Index"=22, "Value"=0.0}, "Y_M"={"Index"=23, "Value"=0.0}, "HORWINDV"={"Index"=26, "Value"=0.0}, "ROOTMOOP1"={"Index"=29, "Value"=0.0}, "ROOTMOOP2"={"Index"=30, "Value"=0.0}, "Blade2PitchPos_rad"={"Index"=32, "Value"=0.0}, "Blade3PitchPos_rad"={"Index"=33, "Value"=0.0}, "ROOTMOOP3"={"Index"=31, "Value"=0.0}, "AVCMSG_SIZE"={"Index"=48, "Value"=0.0}, "INFILE_SIZE "={"Index"=49, "Value"=0.0}, "OUTFILE_SIZE "={"Index"=50, "Value"=0.0}, "FA_ACC"={"Index"=52, "Value"=0.0}, "NUM_BLADES"={"Index"=60, "Value"=0.0}, "BladePitchSetpoint_rad"={"Index"=44, "Value"=0.0}, "TorqueSetpoint_Nm"={"Index"=46, "Value"=0.0}, "OUT_AEROTQ"={"Index"=91, "Value"=0.0}, "Out.RotSpeed "={"Index"=92, "Value"=0.0}, "Out.DEBUG"={"Index"=93, "Value"=0.0}} ("ArrayPairs") -> [w413]
    shift-right: [w380] -> _
    shift-left: T12 {"mainGenPosition (rad)"=0.0, "motorCurrentTorq (Nm)"=0.0, "mainGenVelocity (rad/s)"=0.0, "mainGenStatus"=0, "pitch1Position (rad)"=0.0, "pitch1Velocity (rad/s)"=0.0, "pitch1Status"=0, "pitch2Position (rad)"=0.0, "pitch2Velocity (rad/s)"=0.0, "pitch2Status"=0, "pitch3Position (rad)"=0.0, "pitch3Velocity (rad/s)"=0.0, "pitch3Status"=0, "torqueSensor (Nm)"=0.0, "nacelleAccX (m/s2)"=0.0, "nacelleAccY (m/s2)"=0.0, "nacelleAccZ (m/s2)"=0.0, "pitch1HomeFlag"=FALSE, "pitch2HomeFlag"=FALSE, "pitch3HomeFlag"=FALSE, "towerTopFx (N)"=0.0, "towerTopFy (N)"=0.0, "towerBotMy (Nm)"=0.0} -> [w410]
    tunnel: w44 -> [w407]
    tunnel: w44 -> [w406]
    shift-right: [w365] -> _
    shift-left: T7 {"Enable"=FALSE, "On"=FALSE, "Reset Fault"=FALSE, "Velocity (VFD)"=[]} ("Ctrl Signals") -> [w366]
    i -> [w391]
    stop <- w416 stop-if-true
    # "Main/Control/Execution Loop"
    n137 = node-c288() -> (→"RT Loop Late?":bool, →"RT Loop Duration":i64)  [unwired: 1 in]
    n138 = shared-variable ".\\SharedVars.lvlib\\PitchAxis3State"() -> (w372:T9)  [unwired: 1 in, 1 out]
    n139 = shared-variable ".\\SharedVars.lvlib\\PitchAxis2State"() -> (w373:T9)  [unwired: 1 in, 1 out]
    n140 = shared-variable ".\\SharedVars.lvlib\\PitchAxis1State"() -> (w374:T9)  [unwired: 1 in, 1 out]
    n141 = To Double Precision Float(number=w391) -> (double precision float=w408:dbl)
    n142 = call "ReadIO.vi"("ArrayPairs In"=w413, "PitchAxis1State"=w374, "PitchAxis2State"=w373, "PitchAxis3State"=w372, "IO Signals In"=w410, "ROSCO Params In"=w412, "error in"=w411) -> ("ArrayPairs Out"=w405:T10, "IO Signals Out"=w402:T12, "ROSCO Params Out"=w404:T14, "Torque RAW (V)"=→"Torque RAW (V)":dbl, "error out"=w403:errorcluster)  [unwired: 4 in]
    n143 = Multiply(x=w408, y=w407) -> (x*y=w379:dbl)
    "cRio Time(s)" <- w379
    n144 = call "AssignStatus_v2.vi"("Time (s)"=w379, "Rosco dt (s)"=w406, "LoopCount"=w391, "Wind Estimator u(t=0) FS"="Wind Est. u(t=0)", "error in (no error)"=w403, "ROSCO Params In"=w404, "IO Signals In"=w402, "ArrayPairs In"=w405) -> ("error out"=w399:errorcluster, "ROSCO Params Out"=w400:T14, "IO Signals Out"=w398:T12, "ArrayPairs Out"=w401:T10)
    n145 = shared-variable ".\\SharedVars.lvlib\\CtrlLoopTime_s"(w379) -> ()  [unwired: 1 in, 1 out]
    n146 = call "CreateSwapArray_v4.vi"("Loop count"=w391, "error in (no error)"=w399, "ROSCO Params"=w400, "IO Signals In"=w398, "ArrayPairs"=w401) -> ("error out"=w394:errorcluster, "ROSCO Params Out"=w395:T14, "IO Signals Out"=w393:T12, "ArrayPairs Out"=w396:T10)  [unwired: 3 in]
    n147 = shared-variable ".\\SharedVars.lvlib\\PitchCtrlMS"() -> (w378:T20)  [unwired: 1 in, 1 out]
    n148 = call "CallRosco_v2.vi"("StopLV"="Stop LabVIEW", "error in (no error)"=w394, "ROSCO Params in"=w395, "IO Signals In"=w393, "ArrayPairs"=w396) -> ("error out"=w392:errorcluster, "ROSCO Params Out"=w375:T14, "IO Signals Out"=w409:T12, "ArrayPairs Out"=w376:T10)  [unwired: 3 in]
    n149 = call "PitchCtrl.vi"("ArrayPairs In"=w376, "IO Signals In"=w409, "ROSCO Params in"=w375, "error in (no error)"=w392, "PitchCtrl"=w378, "Time (s)"=w379, "PitchAxis1State"=w374, "PitchAxis2State"=w373, "PitchAxis3State"=w372) -> ("Pitch setpoint (rad)"=w390:dbl, "ArrayPairs Out"=w389:T10, "IO Signals Out"=w388:T12, "ROSCO Params Out"=w387:T14, "error out"=w386:errorcluster)  [unwired: 6 in]
    n150 = shared-variable ".\\SharedVars.lvlib\\PitchSetpoint_rad"(w390) -> ()  [unwired: 1 in, 1 out]
    n151 = shared-variable ".\\SharedVars.lvlib\\GenCtrlMS"() -> (w377:T19)  [unwired: 1 in, 1 out]
    n152 = shared-variable ".\\SharedVars.lvlib\\FanSetpoint_unit"() -> (w364:dbl[])  [unwired: 1 in, 1 out]
    n153 = call "GenCtrl.vi"("Loop Time (s)"=w379, "Gen Control"=w377, "error in (no error)"=w386, "ROSCO Params in"=w387, "IO Signals In"=w388, "ArrayPairs In"=w389) -> ("error out"=w369:errorcluster, "ROSCO Params Out"=w384:T14, "IO Signals Out"=w380:T12, "ArrayPairs Out"=w385:T10, "Velocity setpoint (rad/s)"=w381:dbl, "Torque setpoint (Nm)"=w382:dbl)
    n154 = shared-variable ".\\SharedVars.lvlib\\GenTorqueSetpoint_Nm"(w382) -> ()  [unwired: 1 in, 1 out]
    n155 = shared-variable ".\\SharedVars.lvlib\\GenVelocitySetpoint_radps"(w381) -> ()  [unwired: 1 in, 1 out]
    n156 = call "PLCCtrl.vi"("Turn Fans On"="Turn Fans On", "Clear Faults"="Clear Faults", "Enable Fans"="Enable Fans", "FanSetpoint_uint"=w364, "Error In"=w369, "Ctrl Signals In"=w366) -> ("Error Out"=w368:errorcluster, "Ctrl Signals Out"=w365:T7)  [unwired: 2 in, 2 out]
    n157 = shared-variable ".\\SharedVars.lvlib\\PLCCtrlSignals"(w365) -> ()  [unwired: 1 in, 1 out]
    n158 = Or(x=w368, y="Stop LabVIEW") -> (x .or. y?=w416:bool)
    n159 = shared-variable ".\\SharedVars.lvlib\\IOSignals"(w380) -> ()  [unwired: 1 in, 1 out]
    n160 = shared-variable ".\\SharedVars.lvlib\\RoscoParams"(w384) -> ()  [unwired: 1 in, 1 out]
    n161 = shared-variable ".\\SharedVars.lvlib\\RoscoPairs"(w385) -> ()  [unwired: 1 in, 1 out]
    n162 = shared-variable ".\\SharedVars.lvlib\\StopLabVIEW"(w416) -> ()  [unwired: 1 in, 1 out]
    n163 = node-c288() -> ()  [unwired: 1 in, 1 out]
  }
  n164 = timed-loop {
    timing: w63 -> [_]
    timing-out: [_] -> w62
    shift-right: [w425] -> _
    shift-left: T9 {"Elmo Operational"=FALSE, "Elmo Warning"=FALSE, "Elmo Fault"=FALSE, "Blade Homed"=FALSE, "Blade Homing"=FALSE, "HomePos (rad)"=0.0} ("Elmo State Cluster In") -> [w433]
    shift-right: [w424] -> _
    shift-left: T9 {"Elmo Operational"=FALSE, "Elmo Warning"=FALSE, "Elmo Fault"=FALSE, "Blade Homed"=FALSE, "Blade Homing"=FALSE, "HomePos (rad)"=0.0} ("Elmo State Cluster In") -> [w431]
    shift-right: [w423] -> _
    shift-left: T9 {"Elmo Operational"=FALSE, "Elmo Warning"=FALSE, "Elmo Fault"=FALSE, "Blade Homed"=FALSE, "Blade Homing"=FALSE, "HomePos (rad)"=0.0} ("Elmo State Cluster In") -> [w429]
    stop <- w450 stop-if-true
    # "TO DO:\nOnly allow home button when OP\nClear homing state when not in OP\nCheck if home pos (zero) remains consitent while drive is on/off and LabVIEW is on/off\nSet setpoint to zero when not homed"
    # "used in ctrl loop"
    # "used in ctrl loop"
    # "used in ctrl loop"
    # "Axis No. 3"
    # "Axis No. 2"
    # "Axis No. 1"
    # "State logic"
    n165 = node-c288() -> (→"State logic late?":bool)  [unwired: 1 in]
    n166 = shared-variable ".\\SharedVars.lvlib\\IOSignals"() -> (w422:T12)  [unwired: 1 in, 1 out]
    n167 = call "AccelnetInterface.vi"("Enable"="Enable Accelnet", "Clear Faults"="Clear Accelnet Faults", "IO Signals"=w422) -> ("Control word"=w445:u16, "Accelnet State"=w449:T21)  [unwired: 7 in]
    "Gen ctrl word" <- w445
    n168 = call "ElmoInterface.vi"("Elmo State Cluster In"=w433, "Axis No."=u32 1, "IO Signals"=w422, "Enable"="Enable Pitch Actuators (x3)", "Clear faults"="Clear Pitch Actuator Faults (x3)", "Home"="Home Blades (x3)") -> ("Elmo State Cluster Out"=w425:T9, "State String"=→"Pitch Axis 1 State":string, "Control word"=w442:u16)  [unwired: 7 in]
    "Pitch axis 1 ctrl word" <- w442
    n169 = call "ElmoInterface.vi"("Elmo State Cluster In"=w431, "Axis No."=u32 2, "IO Signals"=w422, "Enable"="Enable Pitch Actuators (x3)", "Clear faults"="Clear Pitch Actuator Faults (x3)", "Home"="Home Blades (x3)") -> ("Elmo State Cluster Out"=w424:T9, "State String"=→"Pitch Axis 2 State":string, "Control word"=w439:u16)  [unwired: 7 in]
    "Pitch axis 2 ctrl word" <- w439
    n170 = call "ElmoInterface.vi"("Elmo State Cluster In"=w429, "Axis No."=u32 3, "IO Signals"=w422, "Enable"="Enable Pitch Actuators (x3)", "Clear faults"="Clear Pitch Actuator Faults (x3)", "Home"="Home Blades (x3)") -> ("Elmo State Cluster Out"=w423:T9, "State String"=→"Pitch Axis 3 State":string, "Control word"=w438:u16)  [unwired: 7 in]
    "Pitch axis 3 ctrl word" <- w438
    n171 = Unbundle By Name(w449) -> ("State String"=→"Main generator state":string, "Accelnet Warning"=→"Generator Warning":bool, "Accelnet Fault"=→"Generator Fault":bool, "Accelnet Operational"=w440:bool)
    "Generator Operational" <- w440
    n172 = shared-variable "NI-cRIO-9036-01B82934\\EtherCAT Master\\MainGen\\Receive PDO 7 CST-Control word"(w445) -> ()  [unwired: 1 in, 1 out]
    n173 = shared-variable ".\\SharedVars.lvlib\\PitchAxis2State"(w424) -> ()  [unwired: 1 in, 1 out]
    n174 = shared-variable "NI-cRIO-9036-01B82934\\EtherCAT Master\\PitchBlade2\\Outputs-Control word"(w439) -> ()  [unwired: 1 in, 1 out]
    n175 = shared-variable ".\\SharedVars.lvlib\\PitchAxis1State"(w425) -> ()  [unwired: 1 in, 1 out]
    n176 = shared-variable "NI-cRIO-9036-01B82934\\EtherCAT Master\\PitchBlade1\\Outputs-Control word"(w442) -> ()  [unwired: 1 in, 1 out]
    n177 = shared-variable ".\\SharedVars.lvlib\\PitchAxis3State"(w423) -> ()  [unwired: 1 in, 1 out]
    n178 = shared-variable "NI-cRIO-9036-01B82934\\EtherCAT Master\\PitchBlade3\\Outputs-Control word"(w438) -> ()  [unwired: 1 in, 1 out]
    n179 = shared-variable ".\\SharedVars.lvlib\\GeneratorOn"(w440) -> ()  [unwired: 1 in, 1 out]
    n180 = shared-variable ".\\SharedVars.lvlib\\StopLabVIEW"() -> (w450:bool)  [unwired: 1 in, 1 out]
    n181 = node-c288() -> ()  [unwired: 1 in, 1 out]
  }
  n182 = timed-loop {
    timing: w59 -> [_]
    timing-out: [_] -> w58
    tunnel: w56 -> [w497]
    i -> [w491]
    stop <- w498 stop-if-true
    # "Data recording to RT buffer"
    n183 = node-c288() -> (→"FIFO Loop Late?":bool)  [unwired: 1 in]
    n184 = shared-variable ".\\SharedVars.lvlib\\GenCtrlMS"() -> (w471:T19)  [unwired: 1 in, 1 out]
    n185 = shared-variable ".\\SharedVars.lvlib\\PitchCtrlMS"() -> (w470:T20)  [unwired: 1 in, 1 out]
    n186 = shared-variable ".\\SharedVars.lvlib\\RoscoPairs"() -> (w475:T10)  [unwired: 1 in, 1 out]
    n187 = shared-variable ".\\SharedVars.lvlib\\GenTorqueSetpoint_Nm"() -> (w463:dbl)  [unwired: 1 in, 1 out]
    n188 = shared-variable ".\\SharedVars.lvlib\\PitchSetpoint_rad"() -> (w462:dbl)  [unwired: 1 in, 1 out]
    n189 = shared-variable ".\\SharedVars.lvlib\\GenVelocitySetpoint_radps"() -> (w461:dbl)  [unwired: 1 in, 1 out]
    n190 = call "FileWriteTiming.vi"("Loop counter"=w491, "WriteData"="Start / Stop Run") -> ("Write counter"=w490:i32, "Time (s)"=w473:dbl)  [unwired: 8 in]
    n191 = shared-variable ".\\SharedVars.lvlib\\WriteData"("Start / Stop Run") -> ()  [unwired: 1 in, 1 out]
    n192 = shared-variable ".\\SharedVars.lvlib\\IOSignals"() -> (w457:T12)  [unwired: 1 in, 1 out]
    n193 = shared-variable ".\\SharedVars.lvlib\\IOSignals"() -> (w495:T12)  [unwired: 1 in, 1 out]
    n194 = To Double Precision Float(number=w490) -> (double precision float=w496:dbl)
    n195 = Unbundle By Name(w457) -> ("towerBotMy (Nm)"=w454:dbl, "towerTopFx (N)"=w455:dbl, "towerTopFy (N)"=w456:dbl)
    n196 = Unbundle By Name(w495) -> ("mainGenPosition (rad)"=w494:dbl, "mainGenVelocity (rad/s)"=w493:dbl, "motorCurrentTorq (Nm)"=w492:dbl, "mainGenStatus"=w488:u16, "pitch1Position (rad)"=w487:dbl, "pitch1Velocity (rad/s)"=w486:dbl, "pitch1Status"=w484:u16, "pitch2Position (rad)"=w483:dbl, "pitch2Velocity (rad/s)"=w482:dbl, "pitch2Status"=w481:u16, "pitch3Position (rad)"=w479:dbl, "pitch3Velocity (rad/s)"=w478:dbl, "pitch3Status"=w477:u16, "nacelleAccX (m/s2)"=w460:dbl, "nacelleAccY (m/s2)"=w459:dbl, "nacelleAccZ (m/s2)"=w458:dbl)
    n197 = Unbundle By Name(w471) -> ("Generator operating mode"=w469:T2)
    n198 = Unbundle By Name(w470) -> ("Blade pitch operating mode"=w466:T4)
    n199 = Unbundle By Name(w475) -> ("TorqueSetpoint_Nm.Value"=w465:dbl, "BladePitchSetpoint_rad.Value"=w464:dbl)  [unwired: 3 out]
    n200 = To Double Precision Float(number=w469) -> (double precision float=w468:dbl)
    n201 = To Double Precision Float(number=w466) -> (double precision float=w467:dbl)
    n202 = To Double Precision Float(number=w484) -> (double precision float=w485:dbl)
    n203 = To Double Precision Float(number=w481) -> (double precision float=w480:dbl)
    n204 = To Double Precision Float(number=w477) -> (double precision float=w476:dbl)
    n205 = To Double Precision Float(number=w488) -> (double precision float=w489:dbl)
    n206 = Bundle By Name(cluster=T6 {"dataTime_s"=0.0, "dataLoopCounter"=0.0, "genPosition_rad"=0.0, "genSpeed_rad_s"=0.0, "genTorque_Nm"=0.0, "genStatus"=0.0, "accelNacelleAx_m_s2"=0.0, "accelNacelleAy_m_s2"=0.0, "accelNacelleAz_m_s2"=0.0, "pitch1Position_rad"=0.0, "pitch1Velocity_rad_s"=0.0, "pitch1Status"=0.0, "pitch2Position_rad"=0.0, "pitch2Velocity_rad_s"=0.0, "pitch2Status"=0.0, "pitch3Position_rad"=0.0, "pitch3Velocity_rad_s"=0.0, "pitch3Status"=0.0, "torqueSetpointRosco_Nm"=0.0, "pitchSetpointRosco_rad"=0.0, "torqueSetpointActual_Nm"=0.0, "pitchSetpointActual_rad"=0.0, "velocitySetpoint_radps"=0.0, "genUserOpMode"=0.0, "pitchUserOpMode"=0.0, "towerTopFx_N"=0.0, "towerTopFy_N"=0.0, "towerTopFz_N"=0.0, "towerTopMx_Nm"=0.0, "towerTopMy_Nm"=0.0, "towerTopMz_Nm"=0.0, "towerBotMy_Nm"=0.0} ("SwapIn"), "dataTime_s"=w473, "dataLoopCounter"=w496, "genPosition_rad"=w494, "genSpeed_rad_s"=w493, "genTorque_Nm"=w492, "genStatus"=w489, "pitch1Position_rad"=w487, "pitch1Velocity_rad_s"=w486, "pitch1Status"=w485, "pitch2Position_rad"=w483, "pitch2Velocity_rad_s"=w482, "pitch2Status"=w480, "pitch3Position_rad"=w479, "pitch3Velocity_rad_s"=w478, "pitch3Status"=w476, "genUserOpMode"=w468, "pitchUserOpMode"=w467, "torqueSetpointRosco_Nm"=w465, "pitchSetpointRosco_rad"=w464, "torqueSetpointActual_Nm"=w463, "pitchSetpointActual_rad"=w462, "velocitySetpoint_radps"=w461, "accelNacelleAx_m_s2"=w460, "accelNacelleAy_m_s2"=w459, "accelNacelleAz_m_s2"=w458, "towerBotMy_Nm"=w454, "towerTopFx_N"=w455, "towerTopFy_N"=w456) -> (w500:T6)
    n207 = call "FileBuffer.vi"("Write Data"="Start / Stop Run", "FileDataChannel"=w500, "Refnum in"=w497) -> ("dataTime_s"=w472:dbl, "# elements"=→"#RT FIFO":u32)  [unwired: 7 in]
    "Exp. Time MS (s)" <- w472
    n208 = shared-variable ".\\SharedVars.lvlib\\ExpTime_s"(w472) -> ()  [unwired: 1 in, 1 out]
    n209 = shared-variable ".\\SharedVars.lvlib\\StopLabVIEW"() -> (w498:bool)  [unwired: 1 in, 1 out]
    n210 = node-c288() -> ()  [unwired: 1 in, 1 out]
  }
  n211 = while {
    shift-right: [w512] -> _
    shift-left: _ -> [w513]
    shift-right: [w518] -> _
    shift-left: FALSE -> [w519]
    shift-right: [w521] -> w65
    shift-left: errorcluster {"status"=FALSE, "code"=0, "source"=""} ("error out") -> [w520]
    tunnel: "focalC1" -> [w515]
    tunnel: w69 -> [w508]
    tunnel: w56 -> [w516]
    tunnel: w14 -> [w507]
    tunnel: w13 -> [w506]
    stop <- w523 stop-if-true
    # "Access the file system every 200ms, writing buffered data. This ensures that the \"slow\" file system is not accessed too often."
    # "Create directory if doesnt exist"
    # "File access loop (non RT loop, read from RT buffer)"
    n212 = Wait (ms)(milliseconds to wait=u32 200) -> ()  [unwired: 1 out]
    n213 = shared-variable ".\\SharedVars.lvlib\\WriteData"() -> (w509:bool)  [unwired: 1 in, 1 out]
    n214 = call "CheckFIleWriteStatus.vi"("WriteDataButtonVal"=w509, "WritePrevVal"=w519, "Refnum in"=w513, "Base filename"="Base filename", "File path"=path "C:/focal-data") -> ("File Name"=→"Output file Name":string, "Refnum out"=w512:refnum<k34>, "WriteCurrentVal"=w518:bool)  [unwired: 4 in]
    n215 = call "WriteToFile-v2.vi"("Refnum in"=w512, "Group Name"=w515, "IO Names"=w508, "rt fifo"=w516, "Write?"=w509, "error in (no error)"=w520, "ConstNames"=w507, "ConstValues"=w506) -> ("Writing to file"=→"Writing":bool, "error out"=w521:errorcluster)  [unwired: 5 in, 1 out]
    n216 = shared-variable ".\\SharedVars.lvlib\\StopLabVIEW"() -> (w524:bool)  [unwired: 1 in, 1 out]
    n217 = Or(x=w521, y=w524) -> (x .or. y?=w523:bool)
  }
  n218 = while {
    tunnel: w55 -> [w642]
    i -> [w636]
    stop <- w655 stop-if-true
    # "Note: This WE is NOT available in the standard version of ROSCO. Need to add in ROSCO src code."
    # "bytes -> Gb"
    # "TSR = r * omega / u"
    # "MN x rad/s -> MW"
    # "TODO - MAKE THIS AND + HOME"
    # "Note: At e.g. 250ms, a chart history of 500 points equates to 20 of real time"
    # "Display/Graphics Loop (non-RT)"
    n219 = shared-variable ".\\SharedVars.lvlib\\IOSignals"() -> (w532:T12)  [unwired: 1 in, 1 out]
    n220 = shared-variable ".\\SharedVars.lvlib\\PitchAxis1State"() -> (w547:T9)  [unwired: 1 in, 1 out]
    n221 = shared-variable ".\\SharedVars.lvlib\\PitchAxis2State"() -> (w540:T9)  [unwired: 1 in, 1 out]
    n222 = shared-variable ".\\SharedVars.lvlib\\PitchAxis3State"() -> (w533:T9)  [unwired: 1 in, 1 out]
    n223 = shared-variable ".\\SharedVars.lvlib\\GenCtrlFS"() -> (w616:T19)  [unwired: 1 in, 1 out]
    n224 = shared-variable ".\\SharedVars.lvlib\\GenCtrlMS"() -> (w631:T19)  [unwired: 1 in, 1 out]
    n225 = shared-variable ".\\SharedVars.lvlib\\RoscoPairs"() -> (w645:T10)  [unwired: 1 in, 1 out]
    n226 = shared-variable ".\\SharedVars.lvlib\\RoscoParams"() -> (w654:T14)  [unwired: 1 in, 1 out]
    n227 = shared-variable ".\\SharedVars.lvlib\\PitchCtrlMS"() -> (w633:T20)  [unwired: 1 in, 1 out]
    n228 = Tick Count (ms)() -> (millisecond timer value=w643:u32)
    n229 = Wait (ms)(milliseconds to wait=u32 250 ("Period")) -> ()  [unwired: 1 out]
    n230 = Subtract(x=w643, y=w642) -> (x-y=w639:u32)
    n231 = To Double Precision Float(number=w636) -> (double precision float=w637:dbl)
    n232 = To Double Precision Float(number=w639) -> (double precision float=w638:dbl)
    n233 = shared-variable ".\\SharedVars.lvlib\\GeneratorOn"() -> (w598:bool)  [unwired: 1 in, 1 out]
    n234 = Unbundle By Name(w532) -> ("mainGenVelocity (rad/s)"=w579:dbl)
    n235 = Unbundle By Name(w532) -> ("motorCurrentTorq (Nm)"=w595:dbl, "torqueSensor (Nm)"=w600:dbl)
    "Torque Sensor (Nm) - NOT scaled" <- w600
    "MotorCurrentTorq (Nm)" <- w595
    n236 = shared-variable ".\\SharedVars.lvlib\\GenTorqueSetpoint_Nm"() -> (w599:dbl)  [unwired: 1 in, 1 out]
    n237 = shared-variable ".\\SharedVars.lvlib\\MotorDemandTorque_Nm"() -> (→"MotorDemandTorque_Nm":dbl)  [unwired: 1 in, 1 out]
    n238 = shared-variable ".\\SharedVars.lvlib\\PitchSetpoint_rad"() -> (w634:dbl)  [unwired: 1 in, 1 out]
    n239 = Unbundle By Name(w532) -> ("pitch1Position (rad)"=w620:dbl, "pitch2Position (rad)"=w619:dbl, "pitch3Position (rad)"=w618:dbl)
    n240 = Unbundle By Name(w532) -> ("mainGenVelocity (rad/s)"=w607:dbl)
    n241 = shared-variable ".\\SharedVars.lvlib\\GenVelocitySetpoint_radps"() -> (w608:dbl)  [unwired: 1 in, 1 out]
    n242 = shared-variable ".\\SharedVars.lvlib\\PitchAxis1State"() -> (w563:T9)  [unwired: 1 in, 1 out]
    n243 = shared-variable ".\\SharedVars.lvlib\\PitchAxis2State"() -> (w562:T9)  [unwired: 1 in, 1 out]
    n244 = shared-variable ".\\SharedVars.lvlib\\PitchAxis3State"() -> (w561:T9)  [unwired: 1 in, 1 out]
    n245 = shared-variable ".\\SharedVars.lvlib\\RoscoParams"() -> (w581:T14)  [unwired: 1 in, 1 out]
    n246 = Unbundle By Name(w532) -> ("nacelleAccX (m/s2)"=→"nacelleAccX (m/s2)":dbl, "nacelleAccY (m/s2)"=→"nacelleAccY (m/s2)":dbl, "nacelleAccZ (m/s2)"=→"nacelleAccZ (m/s2)":dbl)
    n247 = Unbundle By Name(w532) -> ("towerTopFx (N)"=w531:dbl, "towerTopFy (N)"=w530:dbl, "towerBotMy (Nm)"=w529:dbl)
    n248 = Unbundle By Name(w645) -> ("BladePitchSetpoint_rad.Value"=→"Rosco Pitch Setpoint (rad)":dbl, "TorqueSetpoint_Nm.Value"=→"Rosco Setpoint (Nm) - MS":dbl, "Out.RotSpeed.Value"=→"OUT_ROTSP":dbl, "OUT_AEROTQ.Value"=→"OUT_AEROTQ":dbl)
    n249 = Divide(x=w638, y=1000.0) -> (x/y=→"Graphics Update t (s)":dbl)
    n250 = Unbundle By Name(w547) -> ("Elmo Operational"=→"Axis 1 Operational":bool, "Elmo Warning"=→"Axis 1 Warning":bool, "Elmo Fault"=→"Axis 1 Fault":bool, "Blade Homing"=→"Axis 1 Homing":bool, "Blade Homed"=→"Axis 1 Homed":bool, "HomePos (rad)"=→"Axis 1 HomePos (rad)":dbl)
    n251 = Unbundle By Name(w540) -> ("Elmo Operational"=→"Axis 2 Operational":bool, "Elmo Warning"=→"Axis 2 Warning":bool, "Elmo Fault"=→"Axis 2 Fault":bool, "Blade Homing"=→"Axis 2 Homing":bool, "Blade Homed"=→"Axis 2 Homed":bool, "HomePos (rad)"=→"Axis 2 HomePos (rad)":dbl)
    n252 = Unbundle By Name(w533) -> ("Elmo Operational"=→"Axis 3 Operational":bool, "Elmo Warning"=→"Axis 3 Warning":bool, "Elmo Fault"=→"Axis 3 Fault":bool, "Blade Homing"=→"Axis 3 Homing":bool, "Blade Homed"=→"Axis 3 Homed":bool, "HomePos (rad)"=→"Axis 3 HomePos (rad)":dbl)
    n253 = Unbundle By Name(w616) -> ("Constant velocity setpoint (rpm)"=→"Const. vel setpoint FS (rpm)":dbl, "Ramp target velocity (rpm)"=→"Ramp target vel FS (rpm)":dbl, "Ramp time (s)"=→"Ramp time FS (s)":dbl, "Sine mean (Nm)"=→"Torque sine mean FS (Nm)":dbl, "Sine amp (Nm)"=→"Torque sine amp FS (Nm)":dbl, "Sine period (s)"=→"Torque sine period FS (Nm)":dbl)
    n254 = Unbundle By Name(w654) -> ("avrSWAP"=→"avrSWAP":dbl[], "aviFAIL"=w652:i32, "currentMsg"=→"Rosco Interface Current Message":string, "firstMsg"=→"Rosco Interface First Message":string)
    "aviFAIL" <- w652
    n255 = Divide(x=w638, y=w637) -> (x/y=→"Effective graphics rate (ms)":dbl)
    n256 = Unbundle By Name(w631) -> ("Generator operating mode"=→"Current OP mode":T2, "Constant velocity setpoint (rpm)"=→"Const. vel setpoint MS (rpm)":dbl, "Ramp target velocity (rpm)"=→"Ramp target vel MS (rpm)":dbl, "Ramp time (s)"=→"Ramp time MS (s)":dbl, "Sine mean (Nm)"=→"Torque sine mean MS (Nm)":dbl, "Sine amp (Nm)"=→"Torque sine amp MS (Nm)":dbl, "Sine period (s)"=→"Torque sine period MS (Nm)":dbl)
    n257 = Get Volume Info(11:path "C:/" ("path")) -> (2:w573:i64)  [unwired: 1 in, 5 out]
    n258 = Unbundle By Name(w633) -> ("Constant setpoint (deg)"=→"Current Const. (deg)":dbl, "Blade pitch operating mode"=→"Current OP mode":T4)
    n259 = shared-variable ".\\SharedVars.lvlib\\Const"() -> (w584:T1)  [unwired: 1 in, 1 out]
    n260 = To Double Precision Float(number=w573) -> (double precision float=w572:dbl)
    n261 = case shown="False" w598 {
      frame False {
        n262 = property on="Next Op mode" class="RadioBtnsControl (strict)"("DisabledEnum"=T22."Disabled and Grayed Out" ("Disabled")) -> ()  [unwired: 2 in, 2 out]
        n263 = property on="Enable Accelnet" class="Bool (strict)"("Value"=FALSE ("Enable Accelnet")) -> ()  [unwired: 2 in, 2 out]
        n264 = property on="Next OP mode" class="RadioBtnsControl (strict)"("Value"=GenMode."Velocity: Zero" ("Next OP mode")) -> ()  [unwired: 2 in, 2 out]
      }
      frame True {
        n265 = property on="Next Op mode" class="RadioBtnsControl (strict)"("DisabledEnum"=T22."Enabled" ("Disabled")) -> ()  [unwired: 2 in, 2 out]
      }
    }
    n266 = Divide(x=w572, y=1073741824.0) -> (x/y=w570:dbl)
    "Free GB disk" <- w570
    n267 = Unbundle By Name(w563) -> ("Elmo Operational"=w560:bool, "Blade Homed"=w559:bool)
    n268 = Unbundle By Name(w562) -> ("Elmo Operational"=w558:bool, "Blade Homed"=w557:bool)
    n269 = Unbundle By Name(w561) -> ("Elmo Operational"=w556:bool, "Blade Homed"=w555:bool)
    n270 = Unbundle By Name(w581) -> ("avrSWAP"=w577:dbl[])
    n271 = Not Equal To 0?(x=w652) -> (x != 0?=→"Rosco Failed?":bool)
    n272 = Unbundle By Name(w584) -> ("rotorRadius"=w583:sgl, "scaleFactor"=w578:dbl)
    n273 = case shown="\"Gauges & Scopes Full Scale\", Default" "IndicatorScale" {
      tunnel: w600 -> [w668 w679]
      tunnel: [w673 w679] -> w592
      tunnel: w599 -> [w667 w678]
      tunnel: [w672 w678] -> w593
      tunnel: w595 -> [w666 w677]
      tunnel: [w664 w677] -> w594
      tunnel: w531 -> [w663 w676]
      tunnel: w530 -> [w662 w675]
      tunnel: w529 -> [w656 w674]
      tunnel: [w661 w676] -> w528
      tunnel: [w660 w675] -> w527
      tunnel: [w658 w674] -> w526
      frame "Gauges & Scopes Full Scale", Default {
        w659 = ScalingEnum."Model scale -> Full scale" ("Scale Dir")
        n274 = shared-variable ".\\SharedVars.lvlib\\Const"() -> (w669:T1)  [unwired: 1 in, 1 out]
        n275 = Unbundle By Name(w669) -> ("scaleFactor"=w657:dbl)
        n276 = call "ScaleTorque.vi"("Scale Dir"=w659, "Scale factor"=w657, "Torque (In)"=w666) -> ("Torque (Out)"=w665:dbl)  [unwired: 8 in]
        n277 = call "ScaleTorque.vi"("Scale Dir"=w659, "Scale factor"=w657, "Torque (In)"=w668) -> ("Torque (Out)"=w671:dbl)  [unwired: 8 in]
        n278 = call "ScaleTorque.vi"("Scale Dir"=w659, "Scale factor"=w657, "Torque (In)"=w667) -> ("Torque (Out)"=w670:dbl)  [unwired: 8 in]
        n279 = call "ScaleTorque.vi"("Scale Dir"=w659, "Scale factor"=w657, "Torque (In)"=w656) -> ("Torque (Out)"=w658:dbl)  [unwired: 8 in]
        n280 = call "ScaleForce.vi"("Scale Dir"=w659, "Scale factor"=w657, "Force (In)"=w663) -> ("Force (Out)"=w661:dbl)  [unwired: 8 in]
        n281 = call "ScaleForce.vi"("Scale Dir"=w659, "Scale factor"=w657, "Force (In)"=w662) -> ("Force (Out)"=w660:dbl)  [unwired: 8 in]
        n282 = call "NumBy1E6.vi"("x"=w665) -> ("Mx"=w664:dbl)
        n283 = call "NumBy1E6.vi"("x"=w671) -> ("Mx"=w673:dbl)
        n284 = call "NumBy1E6.vi"("x"=w670) -> ("Mx"=w672:dbl)
      }
      frame "Gauges & Scopes Model Scale" {
      }
    }
    "Torque Setpoint" <- w593
    "Torque Cell" <- w592
    "Fx" <- w528
    "Fy" <- w527
    "towerBotMy" <- w526
    n285 = case shown="\"Gauges & Scopes Full Scale\", Default" "IndicatorScale" {
      tunnel: w608 -> [w682 w687]
      tunnel: w607 -> [w683 w688]
      tunnel: [w681 w688] -> w591
      tunnel: [w680 w687] -> w605
      frame "Gauges & Scopes Full Scale", Default {
        w686 = ScalingEnum."Model scale -> Full scale" ("Scale Dir")
        n286 = shared-variable ".\\SharedVars.lvlib\\Const"() -> (w685:T1)  [unwired: 1 in, 1 out]
        n287 = Unbundle By Name(w685) -> ("scaleFactor"=w684:dbl)
        n288 = call "ScaleRotVel.vi"("Scale Dir"=w686, "Scale factor"=w684, "Rotational Velocity (In)"=w682) -> ("Rotational Velocity (Out)"=w680:dbl)  [unwired: 8 in]
        n289 = call "ScaleRotVel.vi"("Scale Dir"=w686, "Scale factor"=w684, "Rotational Velocity (In)"=w683) -> ("Rotational Velocity (Out)"=w681:dbl)  [unwired: 8 in]
      }
      frame "Gauges & Scopes Model Scale" {
      }
    }
    n290 = call "RadToDeg.vi"("rad"=w620) -> ("deg"=w604:dbl)
    "Pitch Blade 1 (deg)" <- w604
    n291 = call "RadToDeg.vi"("rad"=w619) -> ("deg"=w603:dbl)
    "Pitch Bade 2 (deg)" <- w603
    n292 = call "RadToDeg.vi"("rad"=w618) -> ("deg"=w602:dbl)
    "Pitch Blade 3 (deg)" <- w602
    n293 = call "RadToDeg.vi"("rad"=w634) -> ("deg"=w623:dbl)
    "Pitch Setpoint (deg)" <- w623
    n294 = Greater?(x=w570, y=2.0) -> (0:→"Disk > 2GB free?":bool)
    n295 = Index Array(array=w577, index=199) -> (element=w580:dbl)
    "WE ROSCO" <- w580
    n296 = To Double Precision Float(number=w583) -> (double precision float=w588:dbl)
    n297 = call "ScaleRotVel.vi"("Scale Dir"=ScalingEnum."Model scale -> Full scale", "Scale factor"=w578, "Rotational Velocity (In)"=w579) -> ("Rotational Velocity (Out)"=w575:dbl)  [unwired: 8 in]
    n298 = Multiply(x=w588, y=w575) -> (x*y=w587:dbl)
    n299 = Compound Arithmetic op=AND(w560, w559, w558, w557, w556, w555) -> (w554:bool)
    n300 = Merge Signals(w623, w604, w603, w602) -> (→"Pitch":dynamicdata)
    n301 = Divide(x=w587, y=w580) -> (x/y=w586:dbl)
    n302 = case shown="False" w554 {
      frame False {
        n303 = property on="Next OP mode" class="RadioBtnsControl (strict)"("DisabledEnum"=T22."Disabled and Grayed Out" ("Disabled")) -> ()  [unwired: 2 in, 2 out]
      }
      frame True {
        n304 = property on="Next OP mode" class="RadioBtnsControl (strict)"("DisabledEnum"=T22."Enabled" ("Disabled")) -> ()  [unwired: 2 in, 2 out]
      }
    }
    n305 = Merge Signals(w586) -> (→"TSR":dynamicdata)
    n306 = call "RadpsToRPM.vi"("radps"=w591) -> ("rpm"=w622:dbl)
    "Actual Speed MS (rpm)" <- w622
    n307 = call "RadpsToRPM.vi"("radps"=w605) -> ("rpm"=w606:dbl)
    "Speed Setpoint (rpm)" <- w606
    n308 = Compound Arithmetic op=MULTIPLY(w591, w592) -> (→"Power (MW)":dbl)
    n309 = Merge Signals(w606, w622) -> (w621:dynamicdata)
    n310 = Merge Signals(w593, w592, w594, w528) -> (→"Rotor Loads":dynamicdata)
    n311 = Merge Signals(w528, w527, w526) -> (→"TSR 2":dynamicdata)
    n312 = Merge Signals(w621) -> (→"Generator Speed":dynamicdata)
    n313 = shared-variable ".\\SharedVars.lvlib\\StopLabVIEW"() -> (w655:bool)  [unwired: 1 in, 1 out]
  }
  n314 = node-c288(w58) -> ()  [unwired: 1 out]
  n315 = node-c288(w5) -> ()  [unwired: 1 out]
  n316 = node-c288(w62) -> ()  [unwired: 1 out]
  n317 = node-c288(w51) -> ()  [unwired: 1 out]
  n318 = node-c288(w42) -> ()  [unwired: 1 out]
  n319 = call <vilib>:"Simple Error Handler.vi"("error in (no error)"=w49) -> ()  [unwired: 4 in, 5 out]
  n320 = call <vilib>:"Simple Error Handler.vi"("error in (no error)"=w65) -> ()  [unwired: 4 in, 5 out]
  "Setpoints" <- w37
